vi "EOL Manual Controls.vi"(11 "main thread cluster":T1={"Application Status"="", "Switch Output Array"=[], "Switch Value Configuration"=[], "NVH Configuration"={"NVH Station?"=FALSE, "nvh app instance path"="", "NVH_ErrorMessages sv url"="", "NVH_Inputs sv url"="", "NVH_MotionNumber sv url"="", "NVH_Outputs sv url"="", "NVH_PartNumber sv url"="", "NVH_PartNumber_Echo sv url"="", "NVH_SerialNumber sv url"="", "NVH_AmbientTempF sv url"=""}, "rs232 port map"={"PMAC"="", "PS Port"="", "LVDT Unit"="", "RS232"=""}, "ethernet address map"={"LVDT 1 Unit"="172.17.53.143", "LVDT Unit 1 port"=0}, "paths"={"Base Path"=path "", "system error log path"=path "", "Error Table Path"=path "C/Labview Code/System/Error Table", "Store errors log path"=path "C/Labview Code/System/Error Table", "data bytes log path"=path "C/Labview Code/System/Error Table", "network path"=path "C/Labview Code/System/Error Table"}, "Station Index"=0, "Store Data"={"Motion Data Array"=[], "Error Table"=[], "Sun Shade Close Force Limits"={"Overall Min"=0.0, "Overall Max"=0.0, "Avg Min"=0.0, "Avg Max"=0.0, "Truncation Start"=0.0, "Truncation End"=0.0, "Variance"=0.0, "Check Noise"=FALSE}, "Sun Shade Open Force Limits"={"Overall Min"=0.0, "Overall Max"=0.0, "Avg Min"=0.0, "Avg Max"=0.0, "Truncation Start"=0.0, "Truncation End"=0.0, "Variance"=0.0, "Check Noise"=FALSE}, "Sunshade Open Data"=[], "Sunshade Close Data"=[], "Module Info"={"Serial Number"="", "Pallet Number"="", "Sunshade Color"="", "Inalfa Part Number"="", "Customer Number"=""}, "Sunsahde Close Raw Data"=[], "Sunshade Open Raw Data"=[], "Software Version"=[], "Constant Version"=[], "Hardware Version"=[], "Inalfa Part Number ECU"=[], "LVDT Data"=[], "Communication Line 1"=[], "Communication Line 2"=[], "Anti Pinch Force"=[], "Cycle Time"="", "Anti Pinch Vent Force"=[], "iGPS LVDT Data"=[], "data bytes log"=""}, "D in map"={"Abort Test"=enum."Dev2/port2/line6", "Start Test"=enum."Dev2/port2/line6"}, "DO Task"="station 1 dio", "ctl refs"={"Start Test"=refnum, "Abort Test"=refnum, "Manual Control"=refnum, "Route to Repair"=refnum, "Waveform Graph"=refnum, "Motion Data"=refnum, "all station status"=refnum, "Individual Station Status"=refnum, "exit program"=refnum, "Sunshade Servo Data Open"=refnum, "Sunshade Servo Data Close"=refnum, "Red-Rabbit Mode"=refnum, "Direct Manual Ctrl"=refnum}, "misc station config"={"Station Name"="", "is AT station?"=FALSE, "is audit station?"=FALSE, "power supply type"=enum."GENser", "use alt China TP2 LVDT Logic Seq"=FALSE, "hmi operator abort timeout"=0, "dump all analog values even if pass"=FALSE, "debug log pre-filter ap stream bytes"=FALSE, "use separate lvdt x and z extend tags"=FALSE, "is print"=FALSE}, "ethernet tcp refs"={"LVDT Unit"=refnum}, "Sunshade Barcode Scan"={"Sunshade Number 2"="", "Sunshade Number 1"="", "Keyence tuning bank idx"=0}, "AP Test Data"={"Raw Sunshade AP Data"="", "Raw Glass AP Data"="", "PMAC Read Counter"=0.0, "Database AP Data"=[]}, "Motion Status"={"hmi operator abort start time"=0, "Current Data Index"=0, "Analog Data"=[], "Motor Position Hex"=0, "Messages Index"=0, "Last Bytes"=[], "Current Hall Position"=0, "Motion Stop Timer"=0, "Position Test"=enum."Not Tested", "Noise Test"=enum."Not Tested", "motion stop check initialized"=FALSE, "remote sense enabled"=FALSE, "Motion"=enum."Glass Teach"}, "LVDT Status"={"LVDT's stored config"=[], "lvdt precision"={"truncate instead of rounding"=FALSE, "decimal places"=0}}, "Sequence State"={"Step Description"="", "Cycle Start Time"=0, "Step Data String"="", "Pass?"=FALSE, "Seqence"=[], "Active Step"=0, "Testing?"=FALSE, "Red-Rabbit Mode"=FALSE, "route-to-repair mode"=FALSE, "NVH Status"={"Restart IRQ Counter"=0, "NVH Test Needed?"=FALSE, "NVH Test Running?"=FALSE}, "Present (s)"=0.0, "Hold Mode?"=FALSE, "Hold?"=FALSE, "Rx Invalid?"=FALSE}, "misc status"={"delay start time (ticks)"=0, "In Vehicle Mode?"=FALSE, "Diag Mode?"=FALSE, "Serial Port Configured?"=FALSE, "PS Voltage"=0.0, "Diag Serial Port"="", "Part Setup"={"Communication Type"=enum."None", "Send Messages to"=enum."Glass", "RAP Signal"=enum."High", "Motor Type"=enum."Smart Motor", "NVH Part Number"=0, "Turn Off Timer"=0, "Part Type"=""}, "Part History Number"="", "Plant Number"=0, "AP Data Type"=enum."91/61", "Real Rollo?"=FALSE}, "NVH Operator?"=FALSE, "NVH Pass?"=FALSE, "Operator Pass?"=FALSE, "Operator Action?"=FALSE, "Noise Source"=0, "USBHandle"=0, "PeakInfo"="", "PeakNumber"=0, "NVH Motion Steps"=[], "Second Check?"=FALSE, "Decibel data"=[], "Direct Control Info"={"EnableStopOnHome"=FALSE, "EnableStopOnPos"=FALSE, "TeachEvent"=FALSE, "open offset"=0, "close offset"=0, "Derect control"=FALSE, "set position"=[], "teach pass "=FALSE, "Drift offsets"=[], "Hall Positions"=[]}, "manual control(direct)"=FALSE, "LIN INFO"={"Toolkit Type"=enum."Inalfa LIN", "NAD"=36, "Inalfa LIN"={"Master Frame(3C)"="", "Slave Frame(3D)"="NIXNET_exampleLDF", "Request Schedule"="NIXNET_exampleLDF", "Response Schedule"="CEMLIN3DiagResponseSchedule\nSPA3414_ConfigurationsCMAGeely_CEMCALYPSOSDB34XX0Cfg_LIN3_190709_", "Frame Write SCU"="", "Frame Read SCU"="", "LIN Name"=""}, "ADCS LIN"={"Port"="MasterReq\nSPA3414_ConfigurationsCMAGeely_CEMCALYPSOSDB34XX0Cfg_LIN3_190709_", "HW select"=0, "XNET Cluster"="SlaveResp\nSPA3414_ConfigurationsCMAGeely_CEMCALYPSOSDB34XX0Cfg_LIN3_190709_", "ByteCmd Path"=path "C/Labview Code/System/ByteCmdConfig.txt"}, "TS LIN"={"ref info"=refnum, "LIN Channel"=0, "ByteCmd Path"=path "C/Labview Code/System/ByteCmdConfig.txt"}}, "Config Info"=variant} {"LIN INFO"."NAD" format="%.0x"; "LIN INFO"."ADCS LIN"."HW select" items=["NI-XNET", "NI-CAN"]; "LVDT Status"."LVDT's stored config"."Lower Limit" format="%.2f"; "LVDT Status"."LVDT's stored config"."Upper Limit" format="%.2f"; "Store Data"."Sun Shade Open Force Limits"."Variance" format="%.2g"; "Store Data"."Sun Shade Open Force Limits"."Truncation End" format="%.2g"; "Store Data"."Sun Shade Open Force Limits"."Truncation Start" format="%.2g"; "Store Data"."Sun Shade Open Force Limits"."Avg Max" format="%.2g"; "Store Data"."Sun Shade Open Force Limits"."Avg Min" format="%.2g"; "Store Data"."Sun Shade Open Force Limits"."Overall Max" format="%.2g"; "Store Data"."Sun Shade Open Force Limits"."Overall Min" format="%.2g"; "Store Data"."Sun Shade Close Force Limits"."Variance" format="%.2g"; "Store Data"."Sun Shade Close Force Limits"."Truncation End" format="%.2g"; "Store Data"."Sun Shade Close Force Limits"."Truncation Start" format="%.2g"; "Store Data"."Sun Shade Close Force Limits"."Avg Max" format="%.2g"; "Store Data"."Sun Shade Close Force Limits"."Avg Min" format="%.2g"; "Store Data"."Sun Shade Close Force Limits"."Overall Max" format="%.2g"; "Store Data"."Sun Shade Close Force Limits"."Overall Min" format="%.2g"; "Store Data"."Motion Data Array"."Motion Data Limits"."LIN Msg"."Msg" format="%02x"; "Store Data"."Motion Data Array"."Motion Data Limits"."LIN Msg"."ID" format="%02x"}) -> (3 "main thread cluster out":T1={"Application Status"="", "Switch Output Array"=[], "Switch Value Configuration"=[], "NVH Configuration"={"NVH Station?"=FALSE, "nvh app instance path"="", "NVH_ErrorMessages sv url"="", "NVH_Inputs sv url"="", "NVH_MotionNumber sv url"="", "NVH_Outputs sv url"="", "NVH_PartNumber sv url"="", "NVH_PartNumber_Echo sv url"="", "NVH_SerialNumber sv url"="", "NVH_AmbientTempF sv url"=""}, "rs232 port map"={"PMAC"="", "PS Port"="", "LVDT Unit"="", "RS232"=""}, "ethernet address map"={"LVDT 1 Unit"="172.17.53.143", "LVDT Unit 1 port"=0}, "paths"={"Base Path"=path "", "system error log path"=path "", "Error Table Path"=path "C/Labview Code/System/Error Table", "Store errors log path"=path "C/Labview Code/System/Error Table", "data bytes log path"=path "C/Labview Code/System/Error Table", "network path"=path "C/Labview Code/System/Error Table"}, "Station Index"=0, "Store Data"={"Motion Data Array"=[], "Error Table"=[], "Sun Shade Close Force Limits"={"Overall Min"=0.0, "Overall Max"=0.0, "Avg Min"=0.0, "Avg Max"=0.0, "Truncation Start"=0.0, "Truncation End"=0.0, "Variance"=0.0, "Check Noise"=FALSE}, "Sun Shade Open Force Limits"={"Overall Min"=0.0, "Overall Max"=0.0, "Avg Min"=0.0, "Avg Max"=0.0, "Truncation Start"=0.0, "Truncation End"=0.0, "Variance"=0.0, "Check Noise"=FALSE}, "Sunshade Open Data"=[], "Sunshade Close Data"=[], "Module Info"={"Serial Number"="", "Pallet Number"="", "Sunshade Color"="", "Inalfa Part Number"="", "Customer Number"=""}, "Sunsahde Close Raw Data"=[], "Sunshade Open Raw Data"=[], "Software Version"=[], "Constant Version"=[], "Hardware Version"=[], "Inalfa Part Number ECU"=[], "LVDT Data"=[], "Communication Line 1"=[], "Communication Line 2"=[], "Anti Pinch Force"=[], "Cycle Time"="", "Anti Pinch Vent Force"=[], "iGPS LVDT Data"=[], "data bytes log"=""}, "D in map"={"Abort Test"=enum."Dev2/port2/line6", "Start Test"=enum."Dev2/port2/line6"}, "DO Task"="station 1 dio", "ctl refs"={"Start Test"=refnum, "Abort Test"=refnum, "Manual Control"=refnum, "Route to Repair"=refnum, "Waveform Graph"=refnum, "Motion Data"=refnum, "all station status"=refnum, "Individual Station Status"=refnum, "exit program"=refnum, "Sunshade Servo Data Open"=refnum, "Sunshade Servo Data Close"=refnum, "Red-Rabbit Mode"=refnum, "Direct Manual Ctrl"=refnum}, "misc station config"={"Station Name"="", "is AT station?"=FALSE, "is audit station?"=FALSE, "power supply type"=enum."GENser", "use alt China TP2 LVDT Logic Seq"=FALSE, "hmi operator abort timeout"=0, "dump all analog values even if pass"=FALSE, "debug log pre-filter ap stream bytes"=FALSE, "use separate lvdt x and z extend tags"=FALSE, "is print"=FALSE}, "ethernet tcp refs"={"LVDT Unit"=refnum}, "Sunshade Barcode Scan"={"Sunshade Number 2"="", "Sunshade Number 1"="", "Keyence tuning bank idx"=0}, "AP Test Data"={"Raw Sunshade AP Data"="", "Raw Glass AP Data"="", "PMAC Read Counter"=0.0, "Database AP Data"=[]}, "Motion Status"={"hmi operator abort start time"=0, "Current Data Index"=0, "Analog Data"=[], "Motor Position Hex"=0, "Messages Index"=0, "Last Bytes"=[], "Current Hall Position"=0, "Motion Stop Timer"=0, "Position Test"=enum."Not Tested", "Noise Test"=enum."Not Tested", "motion stop check initialized"=FALSE, "remote sense enabled"=FALSE, "Motion"=enum."Glass Teach"}, "LVDT Status"={"LVDT's stored config"=[], "lvdt precision"={"truncate instead of rounding"=FALSE, "decimal places"=0}}, "Sequence State"={"Step Description"="", "Cycle Start Time"=0, "Step Data String"="", "Pass?"=FALSE, "Seqence"=[], "Active Step"=0, "Testing?"=FALSE, "Red-Rabbit Mode"=FALSE, "route-to-repair mode"=FALSE, "NVH Status"={"Restart IRQ Counter"=0, "NVH Test Needed?"=FALSE, "NVH Test Running?"=FALSE}, "Present (s)"=0.0, "Hold Mode?"=FALSE, "Hold?"=FALSE, "Rx Invalid?"=FALSE}, "misc status"={"delay start time (ticks)"=0, "In Vehicle Mode?"=FALSE, "Diag Mode?"=FALSE, "Serial Port Configured?"=FALSE, "PS Voltage"=0.0, "Diag Serial Port"="", "Part Setup"={"Communication Type"=enum."None", "Send Messages to"=enum."Glass", "RAP Signal"=enum."High", "Motor Type"=enum."Smart Motor", "NVH Part Number"=0, "Turn Off Timer"=0, "Part Type"=""}, "Part History Number"="", "Plant Number"=0, "AP Data Type"=enum."91/61", "Real Rollo?"=FALSE}, "NVH Operator?"=FALSE, "NVH Pass?"=FALSE, "Operator Pass?"=FALSE, "Operator Action?"=FALSE, "Noise Source"=0, "USBHandle"=0, "PeakInfo"="", "PeakNumber"=0, "NVH Motion Steps"=[], "Second Check?"=FALSE, "Decibel data"=[], "Direct Control Info"={"EnableStopOnHome"=FALSE, "EnableStopOnPos"=FALSE, "TeachEvent"=FALSE, "open offset"=0, "close offset"=0, "Derect control"=FALSE, "set position"=[], "teach pass "=FALSE, "Drift offsets"=[], "Hall Positions"=[]}, "manual control(direct)"=FALSE, "LIN INFO"={"Toolkit Type"=enum."Inalfa LIN", "NAD"=36, "Inalfa LIN"={"Master Frame(3C)"="", "Slave Frame(3D)"="NIXNET_exampleLDF", "Request Schedule"="NIXNET_exampleLDF", "Response Schedule"="CEMLIN3DiagResponseSchedule\nSPA3414_ConfigurationsCMAGeely_CEMCALYPSOSDB34XX0Cfg_LIN3_190709_", "Frame Write SCU"="", "Frame Read SCU"="", "LIN Name"=""}, "ADCS LIN"={"Port"="MasterReq\nSPA3414_ConfigurationsCMAGeely_CEMCALYPSOSDB34XX0Cfg_LIN3_190709_", "HW select"=0, "XNET Cluster"="SlaveResp\nSPA3414_ConfigurationsCMAGeely_CEMCALYPSOSDB34XX0Cfg_LIN3_190709_", "ByteCmd Path"=path "C/Labview Code/System/ByteCmdConfig.txt"}, "TS LIN"={"ref info"=refnum, "LIN Channel"=0, "ByteCmd Path"=path "C/Labview Code/System/ByteCmdConfig.txt"}}, "Config Info"=variant} {"LIN INFO"."NAD" format="%.0x"; "LIN INFO"."ADCS LIN"."HW select" items=["NI-XNET", "NI-CAN"]; "LVDT Status"."LVDT's stored config"."Lower Limit" format="%.2f"; "LVDT Status"."LVDT's stored config"."Upper Limit" format="%.2f"; "Store Data"."Sun Shade Open Force Limits"."Variance" format="%.2g"; "Store Data"."Sun Shade Open Force Limits"."Truncation End" format="%.2g"; "Store Data"."Sun Shade Open Force Limits"."Truncation Start" format="%.2g"; "Store Data"."Sun Shade Open Force Limits"."Avg Max" format="%.2g"; "Store Data"."Sun Shade Open Force Limits"."Avg Min" format="%.2g"; "Store Data"."Sun Shade Open Force Limits"."Overall Max" format="%.2g"; "Store Data"."Sun Shade Open Force Limits"."Overall Min" format="%.2g"; "Store Data"."Sun Shade Close Force Limits"."Variance" format="%.2g"; "Store Data"."Sun Shade Close Force Limits"."Truncation End" format="%.2g"; "Store Data"."Sun Shade Close Force Limits"."Truncation Start" format="%.2g"; "Store Data"."Sun Shade Close Force Limits"."Avg Max" format="%.2g"; "Store Data"."Sun Shade Close Force Limits"."Avg Min" format="%.2g"; "Store Data"."Sun Shade Close Force Limits"."Overall Max" format="%.2g"; "Store Data"."Sun Shade Close Force Limits"."Overall Min" format="%.2g"; "Store Data"."Motion Data Array"."Motion Data Limits"."LIN Msg"."Msg" format="%02x"; "Store Data"."Motion Data Array"."Motion Data Limits"."LIN Msg"."ID" format="%02x"})   [LabVIEW 2018]
uses:
  02.Type Def's/debug io digital io.ctl
  02.Type Def's/EOL Analog Input Control.ctl
  05.UserVI's/type defs/EOL LVDT's Check Controller.ctl
  02.Type Def's/main state cluster.ctl
  02.Type Def's/All Switch Configuration Cluster.ctl
  02.Type Def's/All Motions.ctl
  02.Type Def's/EOL Switch Value Configuration Cluster.ctl
  02.Type Def's/EOL Switch Max Min Check Cluster.ctl
  02.Type Def's/station nvh config.ctl
  02.Type Def's/station rs232 port map.ctl
  02.Type Def's/station ethernet address map.ctl
  02.Type Def's/station paths.ctl
  02.Type Def's/EOL Save Module Test Data Control.ctl
  02.Type Def's/EOL Motion Database Table.ctl
  05.UserVI's/type defs/17x Audit Motion Data Seq Control.ctl
  05.UserVI's/type defs/17x AP Data Type.ctl
  05.UserVI's/type defs/17x Sunshade Limts Seq.ctl
  02.Type Def's/EOL Module Info Control.ctl
  02.Type Def's/station DI map.ctl
  05.UserVI's/type defs/EOL Global Digital Input Control.ctl
  02.Type Def's/control refs.ctl
  02.Type Def's/station motion data indicator.ctl
  02.Type Def's/Screen Motion Data.ctl
  02.Type Def's/Pass Fail Control.ctl
  02.Type Def's/station hmi.ctl
  02.Type Def's/lvdt name val pair.ctl
  02.Type Def's/individual station status.ctl
  02.Type Def's/misc station config.ctl
  05.UserVI's/Lambda Power/power supply types.ctl
  05.UserVI's/LVDT's/lvdt precision.ctl
  02.Type Def's/sequence state.ctl
  05.UserVI's/sequence/type defs/Sequence Info.ctl
  05.UserVI's/type defs/EOL Part Setup.ctl
  02.Type Def's/All Communication Types.ctl
  05.UserVI's/type defs/Communication with Motors.ctl
  05.UserVI's/type defs/RAP Signal Control.ctl
  05.UserVI's/type defs/EOL Motor Type.ctl
  02.Type Def's/station LIN config.ctl
  03.Inalfa LIN/LIN Device.ctl
  <vilib>/CMC.AME/Inalfa ADCS/Ctl'Def/ADCS_LIN info.ctl
  C:/Program Files (x86)/National Instruments/LabVIEW 2018/vi.lib/CMC.AME/Inalfa TS LIN/TOSUN/TSMaster/bin/Interop.TSMasterAPI.dll
  Program Files (x86)/National Instruments/LabVIEW 2018/vi.lib/CMC.AME/Inalfa TS LIN/TOSUN/TSMaster/bin/Interop.TSMasterAPI.dll
  06.Test Loop/Sub'VIs/Type Def's/Config Info.ctl
  03.Inalfa LIN/LIN sequence for self SCU.ctl
  05.UserVI's/type defs/EOL Global Digital Output Cluster Control.ctl
  05.UserVI's/type defs/EOL Global Digital Output Control.ctl
  05.UserVI's/BarCode/typedefs/barcode format params.ctl
  05.UserVI's/BarCode/typedefs/barcode printer types.ctl
  03.Inalfa LIN/LIN show messages.ctl
  <vilib>/Utility/config.llb/Read Key (String).vi
  <vilib>/Utility/config.llb/Write Key (String).vi
  <vilib>/Instr/_visa.llb/VISA Configure Serial Port (Instr).vi
  <vilib>/Utility/file.llb/Write To Spreadsheet File (string).vi
  <vilib>/Utility/file.llb/Read From Spreadsheet File (string).vi
  <vilib>/Utility/config.llb/NI_LVConfig.lvlib
  <resource>/objmgr/daqmx.rc
panel:
  out "错误输出":errorcluster
  in  "Exit":bool
  out "Title":string="Manual Control"
  in  "Tab Control 3":T35(tab)=enum."Barcode Read and Print"
  in  "Sunroof Operation":bool
  in  "Re-Init PS":bool
  out "All Inputs":T36[](array[typedef])=[{"channel name"="Abort Test", "state"=FALSE}, {"channel name"="Start Test", "state"=FALSE}]
  in  "Set Voltage":bool
  in  "Output Voltage":dbl=13.5
  out "Audit Graph":sgl[][](graph)
  in  "Analog Control":T37
  in  "Analog Control 2":T37=enum."Motor Current"
  in  "Analog Control 3":T37=enum."Switch A"
  in  "Color Box 10":u32(colorbox)=16860
  in  "Color Box 11":u32(colorbox)=16711680
  in  "Color Box 12":u32(colorbox)
  in  "Digital Output Array":T36[](array[typedef])=[{"channel name"="Comm Power", "state"=FALSE}, {"channel name"="Switch 1", "state"=FALSE}, {"channel name"="Switch 2", "state"=FALSE}, {"channel name"="Switch 3", "state"=FALSE}, {"channel name"="Switch 4", "state"=FALSE}, {"channel name"="Switch 5", "state"=FALSE}, {"channel name"="Switch 6", "state"=FALSE}, {"channel name"="Glass Analog Switch 1", "state"=FALSE}, {"channel name"="Glass Analog Switch 2", "state"=FALSE}, {"channel name"="Glass Analog Switch 3", "state"=FALSE}, {"channel name"="Glass Analog Switch 4", "state"=FALSE}, {"channel name"="Glass Motor Relay 1", "state"=FALSE}, {"channel name"="Glass Motor Relay 2", "state"=FALSE}, {"channel name"="Sunshade Motor Relay 1", "state"=FALSE}, {"channel name"="Sunshade Motor Relay 2", "state"=FALSE}, {"channel name"="Ignition High", "state"=FALSE}, {"channel name"="Ignition Low", "state"=FALSE}, {"channel name"="Battery", "state"=FALSE}, {"channel name"="Sunshade Analog Switch 1", "state"=FALSE}, {"channel name"="Sunshade Analog Switch 2", "state"=FALSE}, {"channel name"="Sunshade Analog Switch 3", "state"=FALSE}, {"channel name"="Sunshade Analog Switch 4", "state"=FALSE}, {"channel name"="NI LIN", "state"=FALSE}, {"channel name"="RS232 LIN", "state"=FALSE}, {"channel name"="RS232", "state"=FALSE}, {"channel name"="CAN", "state"=FALSE}, {"channel name"="Park/Enable", "state"=FALSE}]
  out "Communications Tab":enum32{"Send Message"}(tab)
  out "Hold？":bool
  in  "Multicolumn Listbox":i32(listbox)
  in  "Part Type":u16(ring) items=["OE", "EX1H", "EX1E"]
  in  "Send Inalfa SCU Message":bool
  in  "Choose Sequence":T38
  out "LIN show Tags":T39(tab)
  in  "Vent Cycles":u16
  in  "Slide Cycles":u16
  out "slide cycle":u16
  out "Software Level":string
  out "Hardware Level":string
  out "Calfile Level":string
  in  "Tx3":u8[][](array[numeric]) format="%02x"
  in  "Tx2":u8[][](array[numeric]) format="%02x"
  in  "Rx2":u8[](array[numeric]) format="%02x"
  in  "Position":u16
  out "glass position":u16
  out "sunshade position":u16
  in  "BYD Teach":string
  out "Recive？":bool
  in  "Send Message":bool
  in  "Message List":i32(listbox)
  out "Toolkit Type":enum16{"Inalfa LIN", "ADCS LIN", "TS LIN"}(ring)=enum."ADCS LIN"
  out "String":string
  out "RSLinx Read Boolean":cluster{"Tag String":string, "Boolean":bool}[](array[cluster])=[{"Tag String"="", "Boolean"=FALSE}, {"Tag String"="", "Boolean"=FALSE}, {"Tag String"="", "Boolean"=FALSE}, {"Tag String"="", "Boolean"=FALSE}, {"Tag String"="", "Boolean"=FALSE}, {"Tag String"="", "Boolean"=FALSE}, {"Tag String"="", "Boolean"=FALSE}, {"Tag String"="", "Boolean"=FALSE}, {"Tag String"="", "Boolean"=FALSE}, {"Tag String"="", "Boolean"=FALSE}, {"Tag String"="", "Boolean"=FALSE}, {"Tag String"="S101.PXI.Signals.Mounting_Bolts.MountBoltSnsr01", "Boolean"=FALSE}, {"Tag String"="S101.PXI.Signals.Mounting_Bolts.MountBoltSnsr02", "Boolean"=FALSE}, {"Tag String"="S101.PXI.Signals.Mounting_Bolts.MountBoltSnsr03", "Boolean"=FALSE}, {"Tag String"="S101.PXI.Signals.Mounting_Bolts.MountBoltSnsr04", "Boolean"=FALSE}, {"Tag String"="S101.PXI.Signals.Mounting_Bolts.MountBoltSnsr05", "Boolean"=FALSE}, {"Tag String"="S101.PXI.Signals.Mounting_Bolts.MountBoltSnsr06", "Boolean"=FALSE}, {"Tag String"="S101.PXI.Signals.Mounting_Bolts.MountBoltSnsr07", "Boolean"=FALSE}, {"Tag String"="S101.PXI.Signals.Mounting_Bolts.MountBoltSnsr08", "Boolean"=FALSE}, {"Tag String"="S101.PXI.Signals.Mounting_Bolts.MountBoltSnsr09", "Boolean"=FALSE}, {"Tag String"="S101.PXI.Signals.Mounting_Bolts.MountBoltSnsr10", "Boolean"=FALSE}, {"Tag String"="S101.PXI.Signals.Mounting_Bolts.MountBoltSnsr11", "Boolean"=FALSE}, {"Tag String"="S101.PXI.Signals.Mounting_Bolts.MountBoltSnsr12", "Boolean"=FALSE}, {"Tag String"="S101.PXI.Signals.Mounting_Bolts.MountBoltSnsr13", "Boolean"=FALSE}, {"Tag String"="S101.PXI.Signals.Mounting_Bolts.MountBoltSnsr14", "Boolean"=FALSE}, {"Tag String"="S101.PXI.Signals.Mounting_Bolts.MountBoltSnsr15", "Boolean"=FALSE}, {"Tag String"="S101.PXI.Signals.Mounting_Bolts.MountBoltSnsr16", "Boolean"=FALSE}, {"Tag String"="S101.PXI.Signals.Mounting_Bolts.MountBoltSnsr17", "Boolean"=FALSE}, {"Tag String"="S101.PXI.Signals.Mounting_Bolts.MountBoltSnsr18", "Boolean"=FALSE}, {"Tag String"="S101.PXI.Signals.Mounting_Bolts.MountBoltSnsr19", "Boolean"=FALSE}, {"Tag String"="S101.PXI.Signals.Mounting_Bolts.MountBoltSnsr20", "Boolean"=FALSE}, {"Tag String"="S101.PXI.Signals.Mounting_Bolts.MountBoltSnsr21", "Boolean"=FALSE}, {"Tag String"="S101.PXI.Signals.StartTest", "Boolean"=FALSE}, {"Tag String"="S101.PXI.Signals.AbortTest", "Boolean"=FALSE}, {"Tag String"="", "Boolean"=FALSE}, {"Tag String"="", "Boolean"=FALSE}, {"Tag String"="S101.PXI.Signals.SoundTestAbort", "Boolean"=FALSE}, {"Tag String"="S101.PXI.Signals.BCData.Print", "Boolean"=FALSE}, {"Tag String"="", "Boolean"=FALSE}, {"Tag String"="", "Boolean"=FALSE}, {"Tag String"="", "Boolean"=FALSE}, {"Tag String"="", "Boolean"=FALSE}]
  out "RSLinx Read String":cluster{"Tag String":string, "String":string}[](array[cluster])=[{"Tag String"="", "String"=""}, {"Tag String"="", "String"="0"}, {"Tag String"="", "String"=""}, {"Tag String"="", "String"=""}, {"Tag String"="", "String"=""}, {"Tag String"="", "String"=""}, {"Tag String"="", "String"=""}, {"Tag String"="", "String"=""}, {"Tag String"="S101.PXI.Signals.PlltData.Sunshade2", "String"=""}, {"Tag String"="S101.PXI.Signals.BCData.SN", "String"="1234"}, {"Tag String"="S101.PXI.Signals.BCData.PN", "String"="1234"}, {"Tag String"="S101.PXI.Signals.BCData.Color", "String"="red"}, {"Tag String"="S101.PXI.Signals.BCData.Model", "String"="1234"}, {"Tag String"="S101.PXI.Signals.BCData.CN", "String"="5678"}, {"Tag String"="S101.PXI.Signals.BCData.PHN", "String"="5678"}]
  in  "RSLinx Write Tag String Array Data":string[](array[string])=["", "", "", "", "", "", "", "", "", "", ""]
  out "RSLinx Write Tag String Array Names":string[](array[string])
  out "RSLinx Write Tag Boolean Array Names":string[](array[string])
  in  "RSLinx Write Tag Boolean Array Data":bool[](array[boolean])=[FALSE, FALSE, FALSE, FALSE, FALSE, FALSE, FALSE, FALSE, FALSE, FALSE]
  in  "Barcode Print Part Type":u16(ring) items=["OE", "EX1H", "EX1E"]
  in  "Barcode Print Part Type":u16(ring) items=["OE", "EX1H", "EX1E"]
  in  "Scan Audit Station Barcode 2 (ss)":bool
  in  "Line Number":u8 max=9
  in  "Customer Name:":string="BMW"
  in  "PHN:":string
  in  "Customer Number:":string="805902507"
  in  "Part Type:":string
  in  "Print Audit St 2D Barcode":bool
  in  "Sunshade Color":string="Reptile Anthraite Black"
  in  "IRS Number:":string="30022369F"
  in  "Serial Number:":string="00103142014"
  in  "Scan Audit Station Barcode":bool
  in  "Scan Station 50 Sunshade Barcode":bool
  in  "TLL/PHN":string="70"
  in  "Color Name":string="REPTILE ANTHRACITE"
  in  "Inalfa Part Number":string="30022369F"
  in  "Module Serial Number":string="00103142014"
  in  "Customer Number":string="805902507"
  in  "Print Station 60 Barcode":bool
  in  "LVDT Part Type":u16(ring) items=["OE", "EX1H", "EX1E"]
  in  "LVDT's Write Preset Data":bool
  in  "LVDT's Read Preset Data":bool
  in  "LVDT's Read Data":bool
  in  "LVDT's Write Data":bool
  in  "LVDT's Limit Array":T22[](array[typedef])=[{"Upper Limit"=1.0, "Lower Limit"=-1.0, "LVDT Name"="LVDT 1", "Check"=FALSE}, {"Upper Limit"=1.0, "Lower Limit"=-1.0, "LVDT Name"="LVDT 2", "Check"=FALSE}, {"Upper Limit"=1.0, "Lower Limit"=-1.0, "LVDT Name"="LVDT 3", "Check"=FALSE}, {"Upper Limit"=1.0, "Lower Limit"=-1.0, "LVDT Name"="LVDT 4", "Check"=FALSE}, {"Upper Limit"=1.0, "Lower Limit"=-1.0, "LVDT Name"="LVDT 5", "Check"=FALSE}, {"Upper Limit"=1.0, "Lower Limit"=-1.0, "LVDT Name"="LVDT 6", "Check"=FALSE}, {"Upper Limit"=1.0, "Lower Limit"=-1.0, "LVDT Name"="LVDT 7", "Check"=FALSE}, {"Upper Limit"=1.0, "Lower Limit"=-1.0, "LVDT Name"="LVDT 8", "Check"=FALSE}, {"Upper Limit"=1.0, "Lower Limit"=-1.0, "LVDT Name"="LVDT 9", "Check"=FALSE}, {"Upper Limit"=1.0, "Lower Limit"=-1.0, "LVDT Name"="LVDT 10", "Check"=FALSE}, {"Upper Limit"=1.0, "Lower Limit"=-1.0, "LVDT Name"="LVDT 11", "Check"=FALSE}, {"Upper Limit"=1.0, "Lower Limit"=-1.0, "LVDT Name"="LVDT 12", "Check"=FALSE}, {"Upper Limit"=1.0, "Lower Limit"=-1.0, "LVDT Name"="LVDT 13", "Check"=FALSE}, {"Upper Limit"=1.0, "Lower Limit"=-1.0, "LVDT Name"="LVDT 14", "Check"=FALSE}, {"Upper Limit"=1.0, "Lower Limit"=-1.0, "LVDT Name"="LVDT 15", "Check"=FALSE}] {"Lower Limit" format="%.2f"; "Upper Limit" format="%.2f"}
  in  "truncate instead of round":bool
  in  "Desired Decimal Points":u8=2
  out "rs232 port map":T7
  out "Reading Count":dbl
  in  "Clear PMAC Buffer":bool
  out "PMAC Reading":string
  in  "Read PMAC":bool
  out "PMAC Reading 2":string
  # "Sunroof Barcode"
  # "Pallet Number"
  # "Part Type"
  # "Application Status"
  # "Current Step"
  # "Cycle Time"
  # "Pass / Fail"
  # "Shade Close"
  # "Actual Data"
  # "Limits"
  # "Avg Current"
  # "Run Time"
  # "Speed"
  # "Noise Test"
  # "Position"
  # "Shade Open"
  # "Actual Data"
  # "Limits"
  # "Avg Current"
  # "Run Time"
  # "Speed"
  # "Noise Test"
  # "Position"
  # "Vent Close"
  # "Actual Data"
  # "Limits"
  # "Avg Current"
  # "Run Time"
  # "Speed"
  # "Noise Test"
  # "Position"
  # "Vent Open"
  # "Actual Data"
  # "Limits"
  # "Avg Current"
  # "Run Time"
  # "Speed"
  # "Noise Test"
  # "Position"
  # "Slide Close"
  # "Actual Data"
  # "Limits"
  # "Avg Current"
  # "Run Time"
  # "Speed"
  # "Noise Test"
  # "Position"
  # "Slide Open"
  # "Actual Data"
  # "Limits"
  # "Avg Current"
  # "Run Time"
  # "Speed"
  # "Noise Test"
  # "Position"
  # "Min"
  # "N"
  # "Min"
  # "Start"
  # "N"
  # "Max"
  # "N"
  # "Max"
  # "N"
  # "End"
  # "Min"
  # "N"
  # "Min"
  # "Start"
  # "N"
  # "Max"
  # "N"
  # "Max"
  # "N"
  # "End"
  # "Min"
  # "Max"
  # "Sunroof Barcode"
  # "Pallet Number"
  # "Part Type"
  # "Application Status"
  # "Current Step"
  # "Cycle Time"
  # "Pass / Fail"
  # "Shade Close"
  # "Actual Data"
  # "Limits"
  # "Avg Current"
  # "Run Time"
  # "Speed"
  # "Noise Test"
  # "Position"
  # "Shade Open"
  # "Actual Data"
  # "Limits"
  # "Avg Current"
  # "Run Time"
  # "Speed"
  # "Noise Test"
  # "Position"
  # "Vent Close"
  # "Actual Data"
  # "Limits"
  # "Avg Current"
  # "Run Time"
  # "Speed"
  # "Noise Test"
  # "Position"
  # "Vent Open"
  # "Actual Data"
  # "Limits"
  # "Avg Current"
  # "Run Time"
  # "Speed"
  # "Noise Test"
  # "Position"
  # "Slide Close"
  # "Actual Data"
  # "Limits"
  # "Avg Current"
  # "Run Time"
  # "Speed"
  # "Noise Test"
  # "Position"
  # "Slide Open"
  # "Actual Data"
  # "Limits"
  # "Avg Current"
  # "Run Time"
  # "Speed"
  # "Noise Test"
  # "Position"
  # "Min"
  # "N"
  # "Min"
  # "Start"
  # "N"
  # "Max"
  # "N"
  # "Max"
  # "N"
  # "End"
  # "Min"
  # "N"
  # "Min"
  # "Start"
  # "N"
  # "Max"
  # "N"
  # "Max"
  # "N"
  # "End"
  # "Min"
  # "Max"
  # "DO"
  # "DI"
  # "Barcode Printing Station"
  # "Audit Station"
  # "LVDT Name"
  # "Current Value"
  # "Preset"
  # "Preset?"
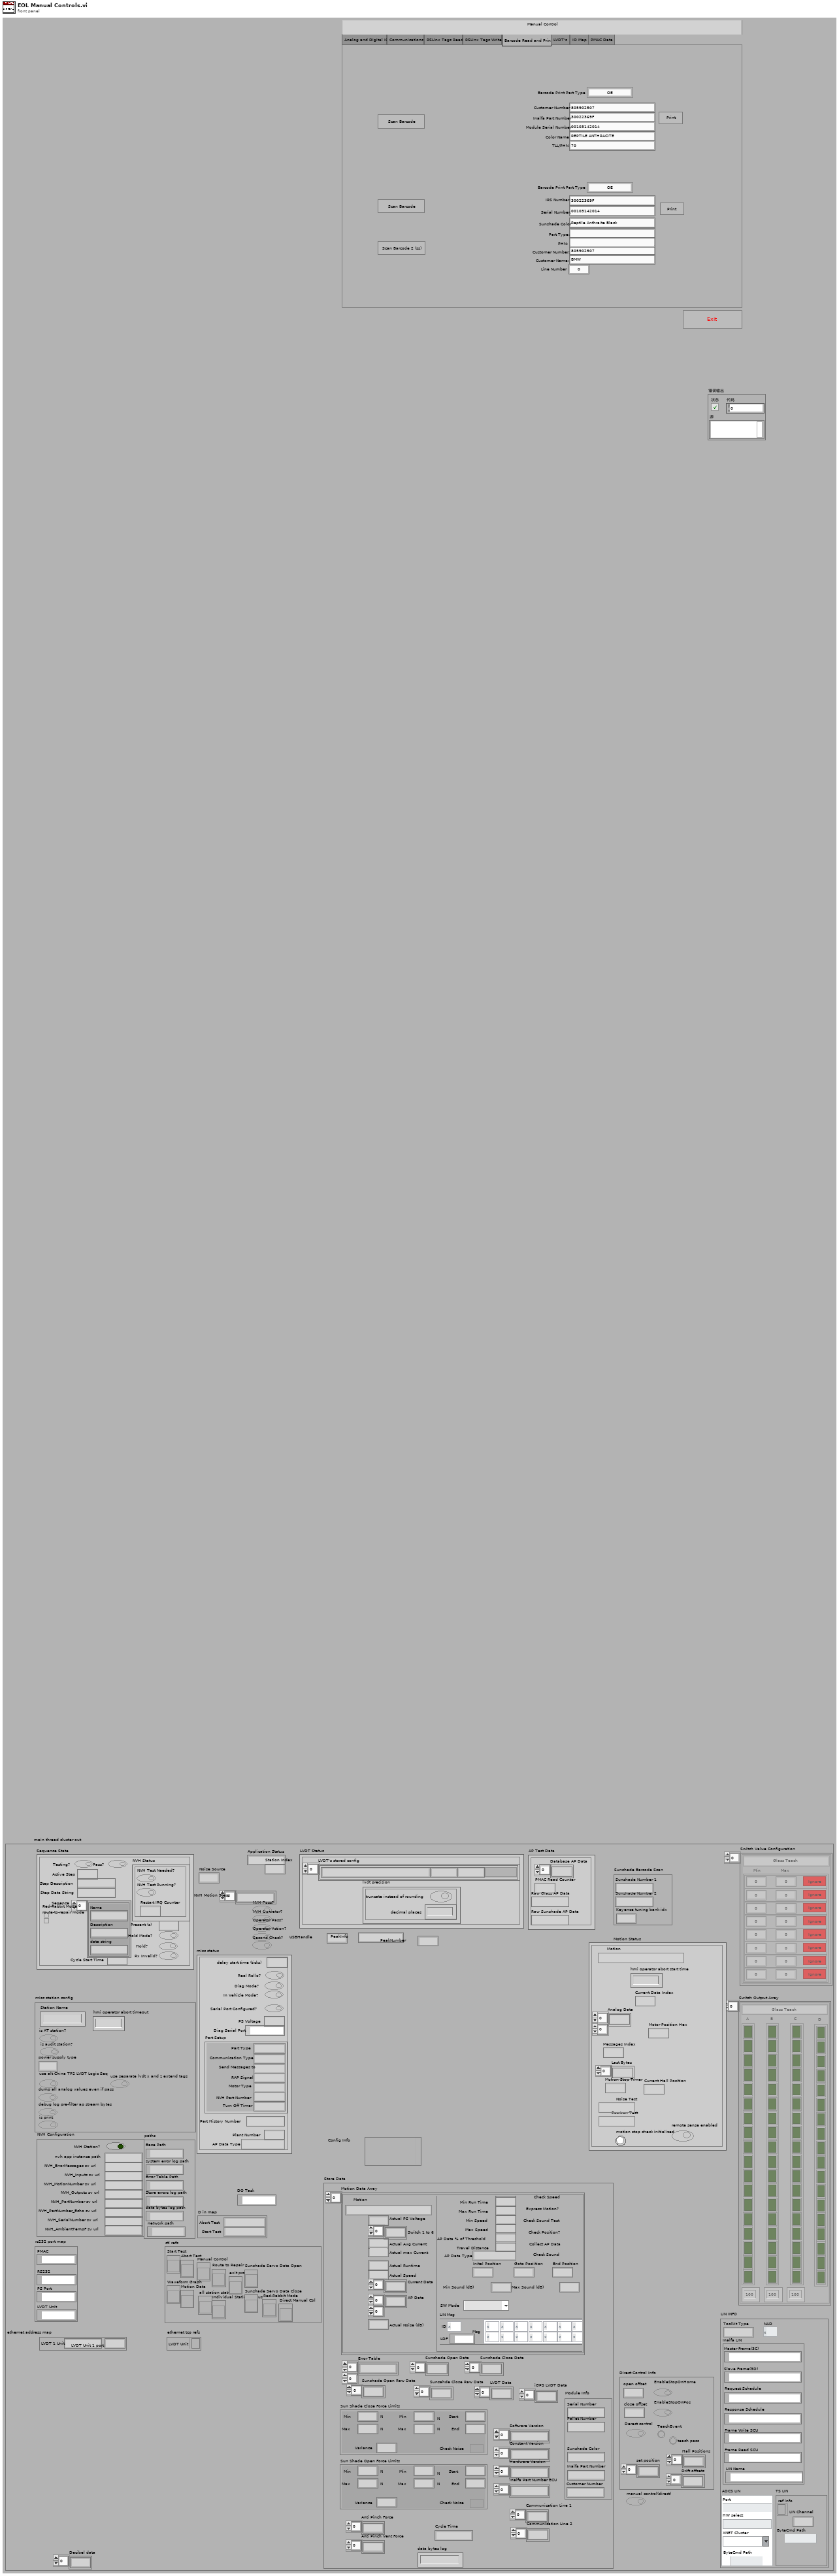
[diagram p1: front panel]
types:
  T1 = typedef "main state cluster.ctl" = cluster{"Application Status":string, "Switch Output Array":T2[], "Switch Value Configuration":T4[], "NVH Configuration":T6, "rs232 port map":T7, "ethernet address map":T8, "paths":T9, "Station Index":i32, "Store Data":T10, "D in map":T16, "DO Task":refnum<k21>, "ctl refs":T18, "misc station config":T19, "ethernet tcp refs":cluster{"LVDT Unit":refnum<k5>}, "Sunshade Barcode Scan":cluster{"Sunshade Number 2":string, "Sunshade Number 1":string, "Keyence tuning bank idx":i32}, "AP Test Data":cluster{"Raw Sunshade AP Data":string, "Raw Glass AP Data":string, "PMAC Read Counter":dbl, "Database AP Data":dbl[]}, "Motion Status":cluster{"hmi operator abort start time":u32, "Current Data Index":i32, "Analog Data":sgl[][], "Motor Position Hex":u16, "Messages Index":u16, "Last Bytes":u8[], "Current Hall Position":i16, "Motion Stop Timer":u32, "Position Test":T21, "Noise Test":T21, "motion stop check initialized":bool, "remote sense enabled":bool, "Motion":T3}, "LVDT Status":cluster{"LVDT's stored config":T22[], "lvdt precision":T23}, "Sequence State":T24, "misc status":cluster{"delay start time (ticks)":u32, "In Vehicle Mode?":bool, "Diag Mode?":bool, "Serial Port Configured?":bool, "PS Voltage":dbl, "Diag Serial Port":refnum<visa-resource-name>, "Part Setup":T26, "Part History Number":string, "Plant Number":u8, "AP Data Type":T13, "Real Rollo?":bool}, "NVH Operator?":bool, "NVH Pass?":bool, "Operator Pass?":bool, "Operator Action?":bool, "Noise Source":u32, "USBHandle":i32, "PeakInfo":string, "PeakNumber":i32, "NVH Motion Steps":string[], "Second Check?":bool, "Decibel data":dbl[], "Direct Control Info":cluster{"EnableStopOnHome":bool, "EnableStopOnPos":bool, "TeachEvent":bool, "open offset":i32, "close offset":i32, "Derect control":bool, "set position":i32[], "teach pass ":bool, "Drift offsets":i32[], "Hall Positions":i32[]}, "manual control(direct)":bool, "LIN INFO":T31, "Config Info":T34}
  T2 = typedef "All Switch Configuration Cluster.ctl" = cluster{"All Motions":T3, "A":bool[], "B":bool[], "C":bool[], "D":bool[], "A activation time (ms)":u32, "B activation time (ms)":u32, "C activation time (ms)":u32}
  T3 = typedef "All Motions.ctl" = enum16{"Glass Teach", "Glass Slide Open", "Glass Slide Close", "Glass Vent Open", "Glass Vent Close", "Sunshade Teach", "Sunshade Open", "Sunshade Close", "Idle", "Sunshade Open 2", "Sunshade Close 2", "Glass Slide Open Sunshade Open", "Glass Slide Open Sunshade Close", "Glass Slide Close Sunshade Open", "Glass Slide Close Sunshade Close", "Glass Vent Open Sunshade Open", "Glass Vent Open Sunshade Close", "Glass Vent Close Sunshade Open", "Glass Vent Close Sunshade Close", "Express Glass Slide Open", "Express Glass Slide Close", "Express Glass Vent Open", "Express Glass Vent Close", "Express Sunshade Open", "Express Sunshade Close", "Express Sunshade Open 2", "Express Sunshade Close 2", "Express Glass Slide Open Sunshade Open", "Express Glass Slide Open Sunshade Close", "Express Glass Slide Close Sunshade Open", "Express Glass Slide Close Sunshade Close", "Express Glass Vent Open Sunshade Open", "Express Glass Vent Open Sunshade Close", "Express Glass Vent Close Sunshade Open", "Express Glass Vent Close Sunshade Close", "Goto Position Glass", "Goto Position Sunshade", "Sunshade Teach 2"}
  T4 = typedef "EOL Switch Value Configuration Cluster.ctl" = cluster{"All Motions":T3, "Array":T5[]}
  T5 = typedef "EOL Switch Max Min Check Cluster.ctl" = cluster{"Min":dbl, "Max":dbl, "Check?":bool}
  T6 = typedef "station nvh config.ctl" = cluster{"NVH Station?":bool, "nvh app instance path":string, "NVH_ErrorMessages sv url":string, "NVH_Inputs sv url":string, "NVH_MotionNumber sv url":string, "NVH_Outputs sv url":string, "NVH_PartNumber sv url":string, "NVH_PartNumber_Echo sv url":string, "NVH_SerialNumber sv url":string, "NVH_AmbientTempF sv url":string}
  T7 = typedef "station rs232 port map.ctl" = cluster{"PMAC":refnum<visa-resource-name>, "PS Port":refnum<visa-resource-name>, "LVDT Unit":refnum<visa-resource-name>, "RS232":refnum<visa-resource-name>}
  T8 = typedef "station ethernet address map.ctl" = cluster{"LVDT 1 Unit":string, "LVDT Unit 1 port":u16}
  T9 = typedef "station paths.ctl" = cluster{"Base Path":path, "system error log path":path, "Error Table Path":path, "Store errors log path":path, "data bytes log path":path, "network path":path}
  T10 = typedef "EOL Save Module Test Data Control.ctl" = cluster{"Motion Data Array":T11[], "Error Table":string[][], "Sun Shade Close Force Limits":T14, "Sun Shade Open Force Limits":T14, "Sunshade Open Data":sgl[], "Sunshade Close Data":sgl[], "Module Info":T15, "Sunsahde Close Raw Data":sgl[], "Sunshade Open Raw Data":sgl[], "Software Version":string[], "Constant Version":string[], "Hardware Version":string[], "Inalfa Part Number ECU":string[], "LVDT Data":sgl[], "Communication Line 1":sgl[], "Communication Line 2":sgl[], "Anti Pinch Force":sgl[], "Cycle Time":string, "Anti Pinch Vent Force":sgl[], "iGPS LVDT Data":sgl[], "data bytes log":string}
  T11 = typedef "EOL Motion Database Table.ctl" = cluster{"Motion":T3, "Actual Avg Current":dbl, "Actual Runtime":dbl, "Actual Speed":dbl, "Current Data":sgl[], "Motion Data Limits":T12, "Switch 1 to 6":dbl[], "Actual PS Voltage":dbl, "AP Data":i16[][], "Actual max Current":dbl, "Actual Noise (dB)":dbl}
  T12 = typedef "17x Audit Motion Data Seq Control.ctl" = cluster{"Power Supply Voltage":dbl, "Min Avg Current":dbl, "Max Avg Current":dbl, "Min Run Time":dbl, "Max Run Time":dbl, "Min Speed":dbl, "Max Speed":dbl, "AP Data % of Threshold":dbl, "Travel Distance":dbl, "AP Data Type":T13, "Check Current":bool, "Check Run Time":bool, "Check Speed":bool, "Express Motion?":bool, "Check Sound Test":bool, "Check Position?":bool, "Collect AP Data":bool, "Inital Position":u16, "End Position":u16, "Goto Posiition":u16, "Max max Current":dbl, "Min max Current":dbl, "Check max Current":bool, "Check Sound":bool, "Min Sound (dB)":dbl, "Max Sound (dB)":dbl, "SW Mode":enum16{"Hard Switch", "Uncond Frame"}, "LIN Msg":cluster{"ID":u8, "Msg":u8[][], "LDF":refnum<k21>}}
  T13 = typedef "17x AP Data Type.ctl" = enum16{"91/61", "92/62", "93/63", "67", "68", "6F", "71", "91 Msg", "92 Msg", "93 Msg", "94 Msg", "HiRain 91", "HiRain 92 Speed", "HiRain 92 HS", "HiRain 92", "HiRain 93", "SnT"}
  T14 = typedef "17x Sunshade Limts Seq.ctl" = cluster{"Overall Min":dbl, "Overall Max":dbl, "Avg Min":dbl, "Avg Max":dbl, "Truncation Start":dbl, "Truncation End":dbl, "Variance":dbl, "Check Noise":bool}
  T15 = typedef "EOL Module Info Control.ctl" = cluster{"Serial Number":string, "Pallet Number":string, "Sunshade Color":string, "Inalfa Part Number":string, "Customer Number":string}
  T16 = typedef "station DI map.ctl" = cluster{"Abort Test":T17, "Start Test":T17}
  T17 = typedef "EOL Global Digital Input Control.ctl" = enum16{"Dev2/port0/line0", "Dev2/port0/line1", "Dev2/port0/line2", "Dev2/port0/line3", "Dev2/port0/line4", "Dev2/port0/line5", "Dev2/port0/line6", "Dev2/port0/line7", "Dev2/port1/line0", "Dev2/port1/line1", "Dev2/port1/line2", "Dev2/port1/line3", "Dev2/port1/line4", "Dev2/port1/line5", "Dev2/port1/line6", "Dev2/port1/line7", "Dev2/port2/line0", "Dev2/port2/line1", "Dev2/port2/line2", "Dev2/port2/line3", "Dev2/port2/line4", "Dev2/port2/line5", "Dev2/port2/line6", "Dev2/port2/line7", "Prerun Start Test", "Prerun Abort Test", "Audit Start Test", "Audit Abort Test", "Dev2/port3/line4", "Dev2/port3/line5", "Breakin Start Test", "Breakin Abort Test", "Not Implemented"}
  T18 = typedef "control refs.ctl" = cluster{"Start Test":refnum<vi>, "Abort Test":refnum<vi>, "Manual Control":refnum<vi>, "Route to Repair":refnum<vi>, "Waveform Graph":refnum<vi>, "Motion Data":refnum<vi>, "all station status":refnum<vi>, "Individual Station Status":refnum<vi>, "exit program":refnum<vi>, "Sunshade Servo Data Open":refnum<vi>, "Sunshade Servo Data Close":refnum<vi>, "Red-Rabbit Mode":refnum<vi>, "Direct Manual Ctrl":refnum<vi>}
  T19 = typedef "misc station config.ctl" = cluster{"Station Name":string, "is AT station?":bool, "is audit station?":bool, "power supply type":T20, "use alt China TP2 LVDT Logic Seq":bool, "hmi operator abort timeout":u32, "dump all analog values even if pass":bool, "debug log pre-filter ap stream bytes":bool, "use separate lvdt x and z extend tags":bool, "is print":bool}
  T20 = typedef "power supply types.ctl" = enum16{"GENser", "ZUPser", "GENeth", "Manual", "ITECH"}
  T21 = typedef "Pass Fail Control.ctl" = enum16{"Not Tested", "Pass", "Fail"}
  T22 = typedef "EOL LVDT's Check Controller.ctl" = cluster{"Upper Limit":dbl, "Lower Limit":dbl, "LVDT Name":string, "Check":bool}
  T23 = typedef "lvdt precision.ctl" = cluster{"truncate instead of rounding":bool, "decimal places":u8}
  T24 = typedef "sequence state.ctl" = cluster{"Step Description":string, "Cycle Start Time":u32, "Step Data String":string, "Pass?":bool, "Seqence":T25[], "Active Step":u8, "Testing?":bool, "Red-Rabbit Mode":bool, "route-to-repair mode":bool, "NVH Status":cluster{"Restart IRQ Counter":u8, "NVH Test Needed?":bool, "NVH Test Running?":bool}, "Present (s)":dbl, "Hold Mode?":bool, "Hold?":bool, "Rx Invalid?":bool}
  T25 = typedef "Sequence Info.ctl" = cluster{"Name":string, "Description":string, "data string":string}
  T26 = typedef "EOL Part Setup.ctl" = cluster{"Communication Type":T27, "Send Messages to":T28, "RAP Signal":T29, "Motor Type":T30, "NVH Part Number":u16, "Turn Off Timer":u16, "Part Type":string}
  T27 = typedef "All Communication Types.ctl" = enum16{"None", "CAN", "RS 232", "RS 232 LIN", "GM LIN", "SnT LIN", "K Line", "Robel CAN", "P42M-Continental", "Inalfa SCU LIN", "Spare 3"}
  T28 = typedef "Communication with Motors.ctl" = enum16{"Glass", "Rollo", "Both"}
  T29 = typedef "RAP Signal Control.ctl" = enum16{"High", "Low", "None"}
  T30 = typedef "EOL Motor Type.ctl" = enum16{"Smart Motor", "Sensor Motor"}
  T31 = typedef "station LIN config.ctl" = cluster{"Toolkit Type":enum16{"Inalfa LIN", "ADCS LIN", "TS LIN"}, "NAD":u8, "Inalfa LIN":T32, "ADCS LIN":T33, "TS LIN":cluster{"ref info":refnum<k24>, "LIN Channel":i32, "ByteCmd Path":path}}
  T32 = typedef "LIN Device.ctl" = cluster{"Master Frame(3C)":refnum<k21>, "Slave Frame(3D)":refnum<k21>, "Request Schedule":refnum<k21>, "Response Schedule":refnum<k21>, "Frame Write SCU":refnum<k21>, "Frame Read SCU":refnum<k21>, "LIN Name":refnum<k21>}
  T33 = typedef "ADCS_LIN info.ctl" = cluster{"Port":string, "HW select":u16, "XNET Cluster":string, "ByteCmd Path":path}
  T34 = typedef "Config Info.ctl" = variant
  T35 = enum32{"Analog and Digital IO", "Communications", "RSLinx Tags Read", "RSLinx Tags Write", "Barcode Read and Print", "LVDT's", "IO Map", "PMAC Data"}
  T36 = typedef "debug io digital io.ctl" = cluster{"channel name":string, "state":bool}
  T37 = typedef "EOL Analog Input Control.ctl" = enum16{"SW PS  Volage", "Switch A", "Switch B", "Switch C", "Motor Voltage", "Motor Current", "ATS"}
  T38 = typedef "LIN sequence for self SCU.ctl" = string
  T39 = enum32{"Blank", "Cycles", "Read Cycles", "Software Level", "Hardware Level", "Calfile Level", "Tx", "Tx and Rx", "Go to position", "Check positions", "BYD Teach"}
  T40 = cluster{"Step Description":string, "Cycle Start Time":u32, "Step Data String":string, "Pass?":bool, "Seqence":cluster{"Name":string, "Description":string, "data string":string}[], "Active Step":u8, "Testing?":bool, "Red-Rabbit Mode":bool, "route-to-repair mode":bool, "NVH Status":cluster{"Restart IRQ Counter":u8, "NVH Test Needed?":bool, "NVH Test Running?":bool}, "Present (s)":dbl, "Hold Mode?":bool, "Hold?":bool, "Rx Invalid?":bool}
  T41 = cluster{"Sequence State in":cluster{"Step Description":string, "Cycle Start Time":u32, "Step Data String":string, "Pass?":bool, "Seqence":cluster{"Name":string, "Description":string, "data string":string}[], "Active Step":u8, "Testing?":bool, "Red-Rabbit Mode":bool, "route-to-repair mode":bool, "NVH Status":cluster{"Restart IRQ Counter":u8, "NVH Test Needed?":bool, "NVH Test Running?":bool}, "Present (s)":dbl, "Hold Mode?":bool, "Hold?":bool, "Rx Invalid?":bool}, "millisecond timer value":u32, "LVDT's Data Array":T22[], "error out":errorcluster}
  T42 = typedef "EOL Global Digital Output Cluster Control.ctl" = cluster{"Status":bool, "Global DO Ch":T43}
  T43 = typedef "EOL Global Digital Output Control.ctl" = enum16{"Battery", "IGN High", "IGN Low", "LIN", "CAN", "Switch 1", "Switch 2", "Switch 3", "Switch 4", "Switch 5", "Switch 6", "Glass Analog Switch 1", "Glass Analog Switch 2", "Glass Analog Switch 3", "Glass Analog Switch 4", "Sunshade Analog Switch 1", "Sunshade Analog Switch 2", "Sunshade Analog Switch 3", "Sunshade Analog Switch 4", "Glass Motor Relay 1", "Glass Motor Relay 2", "Sunshade Motor Relay 1", "Sunshade Motor Relay 2"}
  T44 = enum16{"Init", "Write", "Write All", "Clear All", "Stop"}
  T45 = typedef "barcode format params.ctl" = cluster{"Format String":string, "Print String":string, "Quantity":u8, "printer type":T46, "RS232 Port":string, "IP Address":string, "Ethernet Port":u32}
  T46 = typedef "barcode printer types.ctl" = enum16{"Intermec RS232", "Intermec Ethernet"}
  T47 = typedef "LIN show messages.ctl" = cluster{"Slide Cycles":u16, "Vent Cycles":u16, "String":string, "Tx Bytes":u8[][], "Rx Bytes":u8[], "Only Tx1 Bytes":u8[][], "Go to Position":u16, "Check Glass Position":u16, "Checkgalss":bool, "Check Sunshade Position":u16, "Checksunshade":bool}
  T48 = typedef "ByteCmd.ctl" = cluster{"CMD":string, "Byte":string}
  T49 = typedef "plc comms params.ctl" = cluster{"PLC boolean read Tags":T50, "PLC bool write Tags":T53, "PLC string read Tags":T54, "PLC string write Tags":T55, "use opc":bool, "PLC/OPC Path":string}
  T50 = typedef "station plc read boolean tags.ctl" = cluster{"AT glass position":T51, "AT shade position":T51, "AT in glass wand lower pos":T51, "AT in glass wand up pos":T51, "AT in sunshad wand lower pos":T51, "AT in sunshad wand up pos":T51, "AT in wand home pos":T51, "LVDT's Extended":T51, "bolt check 1":T51, "bolt check 2":T51, "bolt check 3":T51, "bolt check 4":T51, "bolt check 5":T51, "bolt check 6":T51, "bolt check 7":T51, "bolt check 8":T51, "start":T51, "abort":T51, "LVDT's Retracted":T51, "manual barcode print":T51, "ss servo at open":T51, "ss servo at close":T51, "ss servo opening":T51, "ss servo closing":T51, "control slide at home":T51, "control slide left good":T51, "control slide left over stroke":T51, "control slide right good":T51, "control slide right over stroke":T51, "wind deflector high speed pos":T51, "wind deflector low speed pos":T51, "AT VentPMACatHome":T51, "AT VentPMACisExtend":T51, "SS Barcode Scanner Bypassed":T51, "Check Frame Barcode":T51, "Z LVDTs Extended":T51, "NVH Operator Pass":T51, "NVH Operator Fail":T51, "NVH Operator Express Glass Open":T51, "NVH Operator Express Glass Close":T51, "NVH Operator Express Rollo Open01":T51, "NVH Operator Express Rollo Close01":T51, "NVH Operator Express Rollo Open02":T51, "NVH Operator Express Rollo Close02":T51, "NVH Operator Vent Open Noise":T51, "NVH Operator Vent Close Noise":T51, "NVH Operator Sunshade Open Noise":T51, "NVH Operator Sunshade Close Noise":T51, "NVH Operator Glass Open Noise":T51, "NVH Operator Glass Close Noise":T51, "NVH Operator Finish":T51, "NVH Operator Check":T51, "windproof position":T51, "NVH Operator Express Glass vent Open":T51, "NVH Operator Express Glass Vent Close":T51, "NVH Operator Re-do":T51, "AT at vent ATS test pos":T51, "AT at vent ATS Home pos":T51, "Start Adjust LVDT":T51, "Finish Adjust LVDT":T51}
  T51 = typedef "plc path and tag.ctl" = cluster{"Tag Name":string, "Network Path":string, "use opc":bool, "DataSocket Reference":T52}
  T52 = typedef "DataSocket Reference Type.ctl" = cluster{"CWDSLib._DCWDataSocket":refnum<k7>, "CWDSLib._DCWData":refnum<k7>, "OnDataUpdated":u32, "OnStatusUpdated":u32}
  T53 = typedef "station plc write boolean tags.ctl" = cluster{"AT set glass wand lower":T51, "AT set sunshade wand lower":T51, "AT set sunshade wand up":T51, "AT set glass wand up":T51, "AT set wand home pos":T51, "Test Complete Pass":T51, "Test Complete Fail":T51, "Test Started":T51, "Retract LVDT's":T51, "Extend LVDT's":T51, "ss servo open":T51, "ss servo close":T51, "control slide start":T51, "control slide stop":T51, "AT VentPMACHome":T51, "AT VentPMACExtended":T51, "Good Frame Barcode":T51, "Bad Frame Barcode":T51, "Extend Z LVDTS":T51, "NVH SunRoof Moving":T51, "NVH SunRoof Stop":T51, "NVH Pass":T51, "NVH Fail":T51, "NVH Operator Express Glass Opened":T51, "NVH Operator Express Glass Closed":T51, "NVH Operator Express Rollo Opened01":T51, "NVH Operator Express Rollo Closed01":T51, "NVH Operator Express Rollo Opened02":T51, "NVH Operator Pass":T51, "NVH Operator Fail":T51, "NVH Operator Check":T51, "NVH Operator Vent Open Noise":T51, "NVH Operator Vent Close Noise":T51, "NVH Operator Sunshade Open Noise":T51, "NVH Operator Sunshade Close Noise":T51, "NVH Operator Glass Open Noise":T51, "NVH Operator Glass Close Noise":T51, "NVH Operator Finish":T51, "Barcode01 OK":T51, "Barcode02 OK":T51, "AT set to Vent ATS Test Pos":T51, "AT set to Vent ATS Home Pos":T51, "Move LVDT Adjust Station":T51}
  T54 = typedef "station plc read string tags.ctl" = cluster{"Serial Number":T51, "Pallet Number":T51, "Inalfa Part Number":T51, "Shade Color":T51, "Model Type":T51, "Customer Number":T51, "Part History Number":T51, "Shade 1 Barcode":T51, "Shade 2 Barcode":T51, "Manual Serial Number":T51, "Manual Inalfa Part Number":T51, "Manual Shade Color":T51, "Manual Model Type":T51, "Manual Customer Number":T51, "Manual Part History Number":T51}
  T55 = typedef "station plc write string tags.ctl" = cluster{"barcode station error":T51, "error message 0":T51, "error message 1":T51, "error message 2":T51, "error message 3":T51}
  T56 = typedef "NI_LVConfig.lvlib/Config Data RefNum.ctl" = refnum<k1>
  T57 = cluster{"ref info":refnum<k24>, "LIN Channel":i32, "ByteCmd Path":path}
  T58 = cluster{"SW":string, "HW":string, "Cal":string, "RP RF":u8, "Hall":cluster{"Glass":i16, "Rollo":i16}, "Cycle":cluster{"Slide":u16, "Vent":u16}, "Hold？":bool}
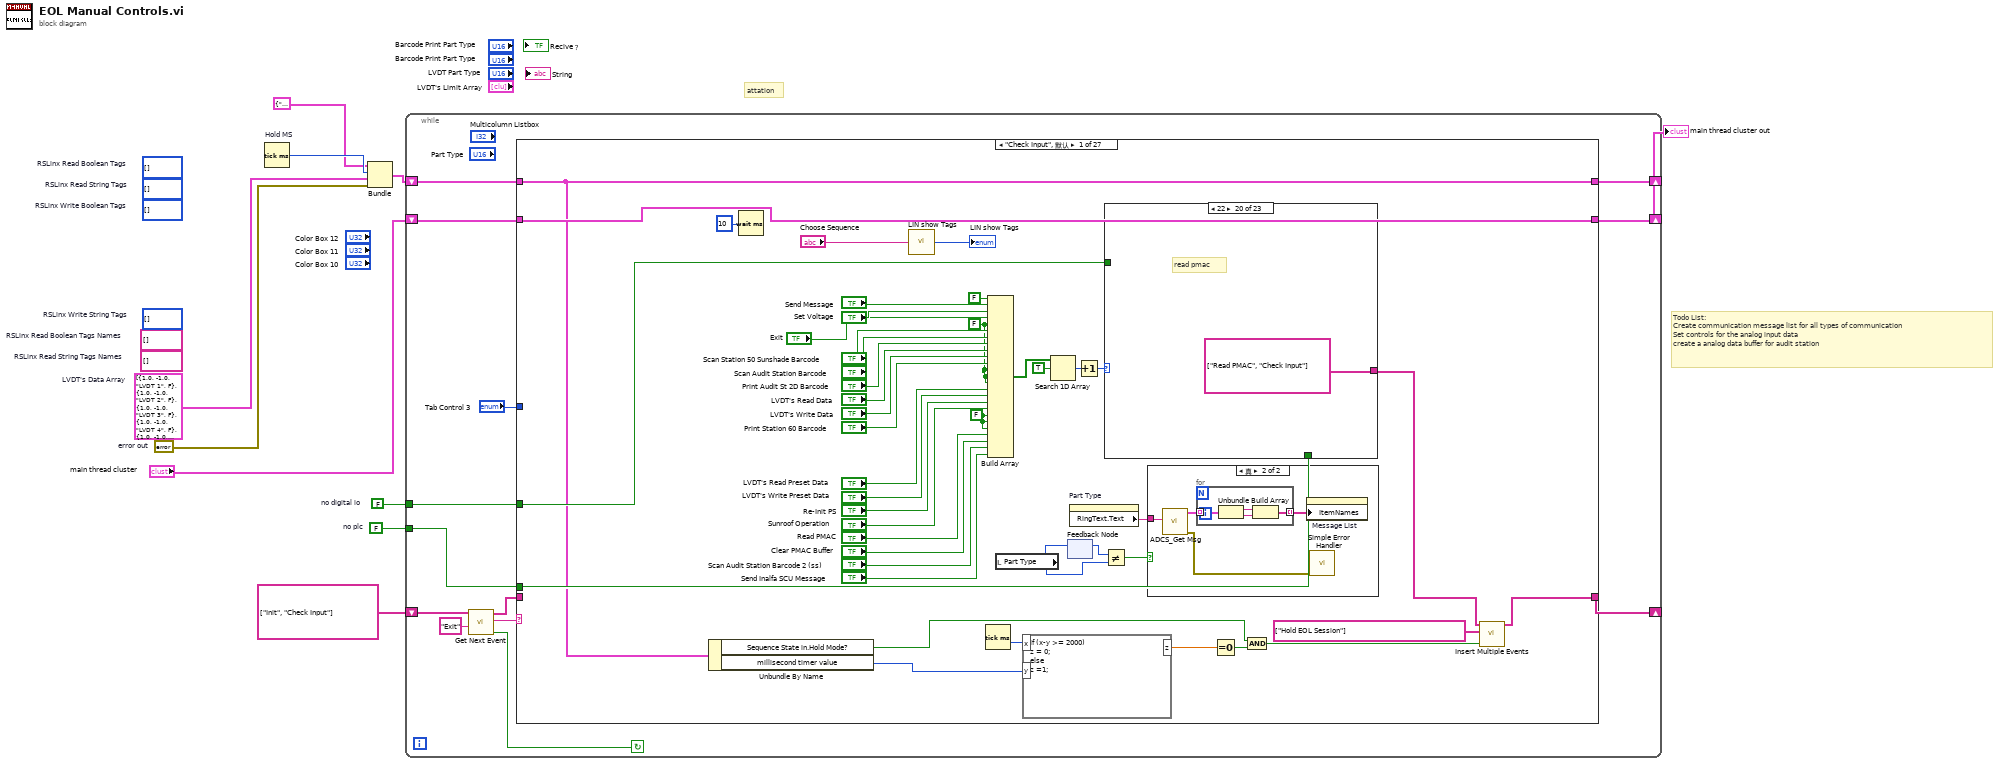
[diagram p0: block diagram]
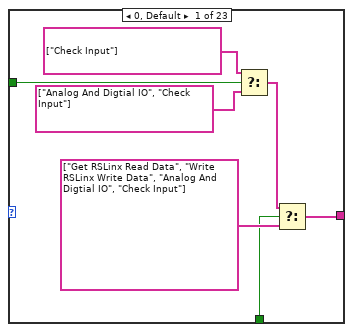
[diagram p3: hidden frame]
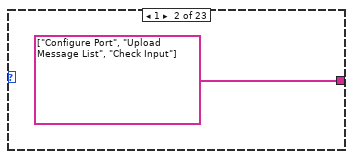
[diagram p4: hidden frame]
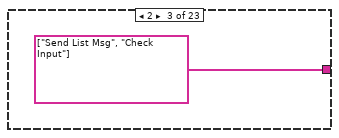
[diagram p5: hidden frame]
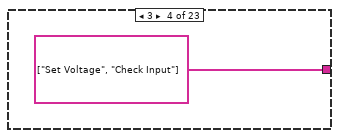
[diagram p6: hidden frame]
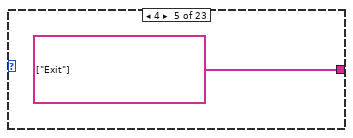
[diagram p7: hidden frame]
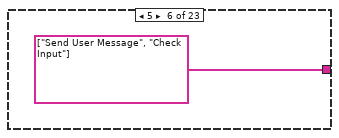
[diagram p8: hidden frame]
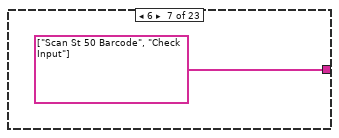
[diagram p9: hidden frame]
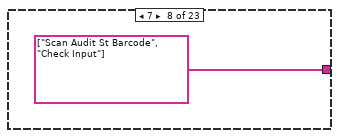
[diagram p10: hidden frame]
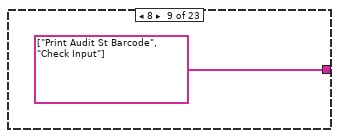
[diagram p11: hidden frame]
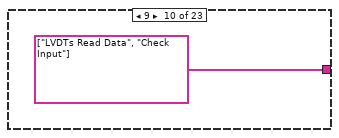
[diagram p12: hidden frame]
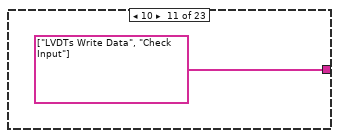
[diagram p13: hidden frame]
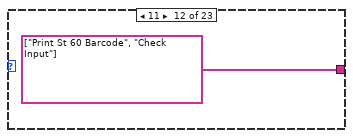
[diagram p14: hidden frame]
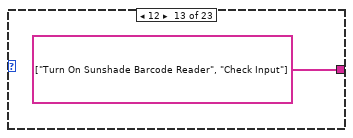
[diagram p15: hidden frame]
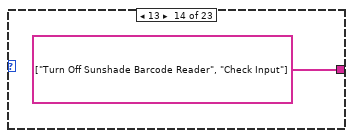
[diagram p16: hidden frame]
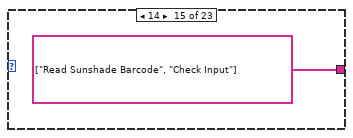
[diagram p17: hidden frame]
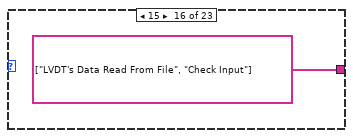
[diagram p18: hidden frame]
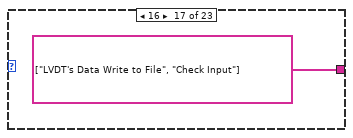
[diagram p19: hidden frame]
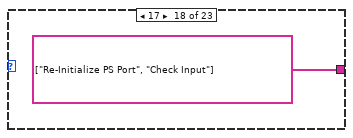
[diagram p20: hidden frame]
diagram:
  w5 = FALSE  # no digital io
  w6 = FALSE  # no plc
  w8 = errorcluster {"status"=FALSE, "code"=0, "source"=""}  # error out
  w9 = T22[] [{"Upper Limit"=1.0, "Lower Limit"=-1.0, "LVDT Name"="LVDT 1", "Check"=FALSE}, {"Upper Limit"=1.0, "Lower Limit"=-1.0, "LVDT Name"="LVDT 2", "Check"=FALSE}, {"Upper Limit"=1.0, "Lower Limit"=-1.0, "LVDT Name"="LVDT 3", "Check"=FALSE}, {"Upper Limit"=1.0, "Lower Limit"=-1.0, "LVDT Name"="LVDT 4", "Check"=FALSE}, {"Upper Limit"=1.0, "Lower Limit"=-1.0, "LVDT Name"="LVDT 5", "Check"=FALSE}, {"Upper Limit"=1.0, "Lower Limit"=-1.0, "LVDT Name"="LVDT 6", "Check"=FALSE}, {"Upper Limit"=1.0, "Lower Limit"=-1.0, "LVDT Name"="LVDT 7", "Check"=FALSE}, {"Upper Limit"=1.0, "Lower Limit"=-1.0, "LVDT Name"="LVDT 8", "Check"=FALSE}, {"Upper Limit"=1.0, "Lower Limit"=-1.0, "LVDT Name"="LVDT 9", "Check"=FALSE}, {"Upper Limit"=1.0, "Lower Limit"=-1.0, "LVDT Name"="LVDT 10", "Check"=FALSE}, {"Upper Limit"=1.0, "Lower Limit"=-1.0, "LVDT Name"="LVDT 11", "Check"=FALSE}, {"Upper Limit"=1.0, "Lower Limit"=-1.0, "LVDT Name"="LVDT 12", "Check"=FALSE}, {"Upper Limit"=1.0, "Lower Limit"=-1.0, "LVDT Name"="LVDT 13", "Check"=FALSE}, {"Upper Limit"=1.0, "Lower Limit"=-1.0, "LVDT Name"="LVDT 14", "Check"=FALSE}]  # LVDT's Data Array
  (unwired) string[] []  # RSLinx Read String Tags Names
  (unwired) string[] []  # RSLinx Read Boolean Tags Names
  (unwired) i32[] []  # RSLinx Write String Tags
  (unwired) i32[] []  # RSLinx Write Boolean Tags
  (unwired) i32[] []  # RSLinx Read String Tags
  (unwired) i32[] []  # RSLinx Read Boolean Tags
  # "attation"
  # "Todo List:\nCreate communication message list for all types of communication \nSet controls for the analog input data\ncreate a analog data buffer for audit station"
  n1 = Tick Count (ms) "Hold MS"() -> (millisecond timer value=w2:u32)
  n2 = Bundle("Sequence State in"=T40 {"Step Description"="", "Cycle Start Time"=0, "Step Data String"="", "Pass?"=FALSE, "Seqence"=[], "Active Step"=0, "Testing?"=FALSE, "Red-Rabbit Mode"=FALSE, "route-to-repair mode"=FALSE, "NVH Status"={"Restart IRQ Counter"=0, "NVH Test Needed?"=FALSE, "NVH Test Running?"=FALSE}, "Present (s)"=0.0, "Hold Mode?"=FALSE, "Hold?"=FALSE, "Rx Invalid?"=FALSE}, "millisecond timer value"=w2, "LVDT's Data Array"=w9, "error out"=w8) -> (w10:T41)  [unwired: 1 in]
  n3 = while {
    shift-right: [w22] -> _
    shift-left: string[] ["Init", "Check Input"] ("event queue out") -> [w14]
    shift-right: [w20] -> _
    shift-left: w10 -> [w21]
    shift-right: [w17] -> w7
    shift-left: "main thread cluster" -> [w13]
    tunnel: w6 -> [w16]
    tunnel: w5 -> [w15]
    stop <- w19 continue-if-true
    n4 = call "Get Next Event.vi"("Exit Event"="Exit", "event queue in"=w14) -> ("Condition (Exit:F)"=w19:bool, "next event"=w23:string, "event queue out"=w12:string[])  [unwired: 3 in]
    n5 = case shown="\"Check Input\", 默认" w23 {
      tunnel: w12 -> [_ w109 w128 w150 w154 w164 w240 w276 w289 w306 w322 w347 w385 w414 w440 w547 w588 w635 w645 w674 w709 w713 _ w722 w734 w745 w763]
      tunnel: [w37 w109 w128 w150 w154 w164 w240 w276 w289 w305 w322 w347 w385 w414 w440 w547 w588 w635 w645 w674 w709 w713 string[] ["Check Input"] ("event queue out") w722 w734 w745 w763] -> w22
      tunnel: w21 -> [w35 w110 w129 w149 w158 w163 w220 w275 w290 w303 w324 w346 w384 w415 w425 w542 w579 w634 w644 w673 w710 w714 w718 w723 w735 w751 w767]
      tunnel: [w35 w110 w129 w149 w158 w163 w220 w275 w290 w303 w324 w346 w384 w412 w424 w546 w578 w634 w644 w673 w710 w714 w718 w723 w735 w751 w767] -> w20
      tunnel: w13 -> [w49 w106 w115 w148 w155 w160 w215 w263 w278 w302 w321 w342 w381 w410 w431 w553 w593 w633 w641 w670 w712 w715 w717 w720 w732 w746 w764]
      tunnel: [w49 w106 w115 w148 w156 w160 w215 w263 w278 w302 w321 w342 w381 w410 w431 w553 w593 w633 w641 w670 w712 w715 w717 w720 w732 w746 w764] -> w17
      tunnel: w16 -> [w48 _ _ _ _ _ _ _ _ _ _ _ _ _ _ _ _ _ _ _ _ _ _ _ _ _ _]
      tunnel: w15 -> [w47 _ _ _ _ _ _ _ _ _ _ _ _ _ _ _ _ _ _ _ _ _ _ w721 w733 _ _]
      tunnel: "Tab Control 3" -> [_ _ _ _ _ w162 _ _ _ _ _ _ _ _ _ _ _ _ _ w672 _ _ _ _ _ _ _]
      frame "Check Input", Default {
        w24 = FALSE ("元素")
        w40 = FALSE ("元素")
        n6 = Unbundle By Name(w35) -> ("Sequence State in.Hold Mode?"=w31:bool, "millisecond timer value"=w33:u32)
        n7 = Wait (ms)(milliseconds to wait=u32 10) -> ()  [unwired: 1 out]
        n8 = call "LIN show Tags.vi"("Choose Sequence"="Choose Sequence") -> ("LIN show Tags"=→"LIN show Tags":T39)  [unwired: 4 in]
        n9 = Tick Count (ms)() -> (millisecond timer value=w34:u32)
        n10 = Build Array(FALSE ("元素"), "Send Message", "Set Voltage", "Exit", w24, "Scan Station 50 Sunshade Barcode", "Scan Audit Station Barcode", "Print Audit St 2D Barcode", "LVDT's Read Data", "LVDT's Write Data", "Print Station 60 Barcode", w24, w24, w24, "LVDT's Read Preset Data", "LVDT's Write Preset Data", "Re-Init PS", "Sunroof Operation", w40, w40, w40, "Read PMAC", "Clear PMAC Buffer", "Scan Audit Station Barcode 2 (ss)", "Send Inalfa SCU Message") -> (w64:bool[])
        n11 = local read "Part Type"() -> (w27:u16)
        n12 = formula code="if (x-y >= 2000) \nz = 0;\nelse\nz =1;"("x"=w34, "y"=w33) -> ("z"=w32:dbl)
        n13 = Search 1D Array(1D array=w64, element=TRUE) -> (index of element=w62:i32)  [unwired: 1 in]
        n14 = feedback #1() -> (w28:u16)  [unwired: 1 in]
        n15 = feedback-in #1(w27) -> ()
        n16 = property on="Part Type" class="Ring (严格)"() -> ("RingText.Text"=w25:string)  [unwired: 2 in, 2 out]
        n17 = Increment(x=w62) -> (x+1=w61:i32)
        n18 = Not Equal?(x=w28, y=w27) -> (x != y?=w26:bool)
        n19 = case shown="22" w61 {
          tunnel: [w80 string[] ["Configure Port", "Upload Message List", "Check Input"] ("event queue out") string[] ["Send List Msg", "Check Input"] ("event queue out") string[] ["Set Voltage", "Check Input"] ("event queue out") string[] ["Exit"] ("event queue out") string[] ["Send User Message", "Check Input"] ("event queue out") string[] ["Scan St 50 Barcode", "Check Input"] ("event queue out") string[] ["Scan Audit St Barcode", "Check Input"] ("event queue out") string[] ["Print Audit St Barcode", "Check Input"] ("event queue out") string[] ["LVDTs Read Data", "Check Input"] ("event queue out") string[] ["LVDTs Write Data", "Check Input"] ("event queue out") string[] ["Print St 60 Barcode", "Check Input"] ("event queue out") string[] ["Turn On Sunshade Barcode Reader", "Check Input"] ("event queue out") string[] ["Turn Off Sunshade Barcode Reader", "Check Input"] ("event queue out") string[] ["Read Sunshade Barcode", "Check Input"] ("event queue out") string[] ["LVDT's Data Read From File", "Check Input"] ("event queue out") string[] ["LVDT's Data Write to File", "Check Input"] ("event queue out") string[] ["Re-Initialize PS Port", "Check Input"] ("event queue out") string[] ["Sunroof Operation", "Check Input"] ("event queue out") string[] ["Read PMAC", "Check Input"] ("event queue out") string[] ["Clear PMAC Buffer", "Check Input"] ("event queue out") string[] ["Scan Audit St Barcode 2", "Check Input"] ("event queue out") string[] ["Send Inalfa SCU Message", "Check Input"] ("event queue out")] -> w38
          tunnel: w48 -> [w81 _ _ _ _ _ _ _ _ _ _ _ _ _ _ _ _ _ _ _ _ _ _]
          tunnel: w47 -> [w77 _ _ _ _ _ _ _ _ _ _ _ _ _ _ _ _ _ _ _ _ _ _]
          frame 0, Default {
            n20 = Select(t=string[] ["Check Input"] ("event queue out"), s=w77, f=string[] ["Analog And Digtial IO", "Check Input"] ("event queue out")) -> (s? t:f=w78:string[])
            n21 = Select(t=w78, s=w81, f=string[] ["Get RSLinx Read Data", "Write RSLinx Write Data", "Analog And Digtial IO", "Check Input"] ("event queue out")) -> (s? t:f=w80:string[])
          }
          frame 1 {
          }
          frame 2 {
          }
          frame 3 {
          }
          frame 4 {
          }
          frame 5 {
          }
          frame 6 {
          }
          frame 7 {
          }
          frame 8 {
          }
          frame 9 {
          }
          frame 10 {
          }
          frame 11 {
          }
          frame 12 {
          }
          frame 13 {
          }
          frame 14 {
          }
          frame 15 {
          }
          frame 16 {
          }
          frame 17 {
          }
          frame 18 {
          }
          frame 22 {
            # "read pmac"
          }
          frame 23 {
            # "clear pmac buffers"
          }
          frame 24 {
          }
          frame 25 {
          }
        }
        n22 = case shown="真" w26 {
          tunnel: w25 -> [_ w71]
          frame False {
          }
          frame True {
            n23 = call <vilib>:"ADCS_Get Msg.vi"("Mode type"=w71) -> ("错误输出"=w68:errorcluster, "LIN Msg"=w70:T48[])  [unwired: 6 in, 2 out]
            n24 = for {
              tunnel: w70 -> [w75] mode=indexing
              tunnel: [w72] -> w69 mode=indexing
              n25 = Unbundle(w75) -> ("CMD"=w74:string, "Byte"=w73:string)
              n26 = Build Array(w74, w73) -> (w72:string[])
            }
            n27 = property on="Message List" class="MCListbox (严格)"("ItemNames"=w69) -> ()  [unwired: 2 in, 2 out]
            n28 = call <vilib>:"Simple Error Handler.vi"("error in (no error)"=w68) -> ()  [unwired: 4 in, 5 out]
          }
        }
        n29 = Equal To 0?(x=w32) -> (x = 0?=w30:bool)
        n30 = And(x=w31, y=w30) -> (x .and. y?=w29:bool)
        n31 = call "Insert Multiple Events.vi"("Insert all? (T)"=w29, "Events to Insert"=string[] ["Hold EOL Session"], "Event queue in"=w38) -> ("Event queue out"=w37:string[])  [unwired: 4 in]
      }
      frame "Sunroof Operation" {
        n32 = Unbundle By Name(w106) -> ("misc station config.Station Name"=w107:string, "Station Index"=w108:i32)
        n33 = Unbundle By Name(w106) -> ("DO Task"=w105:refnum<k21>)
        n34 = call "EOL Manual Sunroof Control.vi"("DO Task"=w105, "station name"=w107, "station idx"=w108) -> ()  [unwired: 9 in]
      }
      frame "Analog And Digtial IO" {
        n35 = Unbundle By Name(w115) -> ("Station Index"=w125:i32, "D in map"=w123:T16)
        n36 = Unbundle By Name(w115) -> ("DO Task"=w114:refnum<k21>)
        n37 = call "EOL All-Station AI Circular Data Buffer.vi"("station idx"=w125, "Mode"=enum16{"Initialize", "Read", "Write"}."Read") -> ("Data Read (Samp-Ro, Ch-Col)"=w126:sgl[][])  [unwired: 9 in]
        n38 = Cluster To Array(cluster=w123) -> (array=w120:T17[])
        n39 = for {
          tunnel: "Digital Output Array" -> [w147] mode=indexing
          tunnel: [w145] -> w112 mode=indexing
          tunnel: T42 {"Status"=FALSE, "Global DO Ch"=enum."Battery"} ("Cluster") -> [w144]
          n40 = Unbundle By Name(w147) -> ("channel name"=w142:string, "state"=w146:bool)
          n41 = Scan From String(input string=w142, default 1=EOL_Global_Digital_Output_Control."Battery" ("Global DO Ch")) -> (output 1=w141:T43)  [unwired: 3 in, 3 out]
          n42 = Bundle By Name(cluster=w144, "Global DO Ch"=w141, "Status"=w146) -> (w145:T42)
        }
        n43 = Index Array(array=w126, index (col) #1="Analog Control", index (col) #2="Analog Control 2", index (col) #3="Analog Control 3") -> (element #1=w130:sgl[], element #2=w131:sgl[], element #3=w132:sgl[])  [unwired: 3 in]
        n44 = Build Array(w130, w131, w132) -> (→"Audit Graph":sgl[][])
        n45 = local read "All Inputs"() -> (w122:T36[])
        n46 = call "EOL Digital Inputs v2.vi"("Digital Inputs Array"=w120, "Mode"=enum16{"Init", "Read", "Read All", "Close"}."Read") -> ("DI Status"=w121:bool[])  [unwired: 7 in, 2 out]
        n47 = Empty Array?(array=w112) -> (empty?=w111:bool)
        n48 = case shown="假" w111 {
          tunnel: w114 -> [w136 _]
          tunnel: w112 -> [w135 _]
          frame False {
            n49 = call "EOL Digital Outputs v3.vi"("task/channels in"=w136, "DO Status"=w135, "Mode"=T44."Write") -> ()  [unwired: 7 in, 2 out]
          }
          frame True {
          }
        }
        n50 = for {
          tunnel: w122 -> [w140] mode=indexing
          tunnel: w121 -> [w138] mode=indexing
          tunnel: [w139] -> w119 mode=indexing
          n51 = Bundle By Name(cluster=w140, "state"=w138) -> (w139:T36)
        }
        "All Inputs" <- w119
      }
      frame "Error" {
      }
      frame "Exit" {
        n52 = Unbundle By Name(w155) -> ("misc status.Diag Serial Port"=w157:refnum<visa-resource-name>)  [unwired: 1 out]
        n53 = VISA Close(VISA resource name=w157) -> (error out=w151:errorcluster)  [unwired: 1 in]
        n54 = call <vilib>:"Clear Errors.vi"("error in (no error)"=w151) -> ()  [unwired: 5 in, 2 out]
        n55 = Bundle By Name(cluster=w155, "misc status.Serial Port Configured?"=FALSE ("Serial Port Configured?")) -> (w156:T1)
        n56 = local write "Communications Tab"(enum32{"Send Message"}."Send Message" ("Communications Tab")) -> ()
      }
      frame "Get RSLinx Read Data" {
        n57 = Unbundle By Name(w160) -> ("Config Info"=w161:T34)
        n58 = call "Config Info Get.vi"("Config Info"=w161) -> ("PLC Comms"=w159:T49)  [unwired: 7 in, 3 out]
        n59 = case shown="\"RSLinx Tags Read\"" w162 {
          tunnel: w159 -> [_ w175]
          frame "Analog and Digital IO", Default {
          }
          frame "RSLinx Tags Read" {
            w166 = errorcluster {"status"=FALSE, "code"=0, "source"=""} ("error out")
            n60 = Unbundle By Name(w175) -> ("PLC boolean read Tags"=w170:T50, "PLC string read Tags"=w173:T54)
            n61 = Cluster To Array(cluster=w170) -> (array=w169:T51[])
            n62 = Cluster To Array(cluster=w173) -> (array=w174:T51[])
            n63 = for {
              tunnel: w169 -> [w178] mode=indexing
              tunnel: [w181] -> w171 mode=indexing
              shift-right: [w177] -> w168
              shift-left: w166 -> [w176]
              n64 = Unbundle By Name(w178) -> ("Tag Name"=w180:string)
              n65 = Empty String/Path?(string/path=w180) -> (empty?=w179:bool)
              n66 = case shown="假" w179 {
                tunnel: w180 -> [w189 _]
                tunnel: [w188 _] -> w181
                tunnel: w178 -> [w185 _]
                tunnel: [w184 w190] -> w177
                tunnel: w176 -> [w183 w190]
                frame False {
                  n67 = Wait Until Next ms Multiple(millisecond multiple=u32 1) -> ()  [unwired: 1 out]
                  n68 = call "plc read bool.vi"("error in"=w183, "addr,tag"=w185) -> ("error out"=w184:errorcluster, "value"=w186:bool)  [unwired: 8 in]
                  n69 = Bundle By Name(cluster=cluster{"Tag String":string, "Boolean":bool} {"Tag String"="", "Boolean"=FALSE} ("Cluster"), "Tag String"=w189, "Boolean"=w186) -> (w188:cluster{"Tag String":string, "Boolean":bool})
                }
                frame True {
                }
              }
            }
            "RSLinx Read Boolean" <- w171
            n70 = for {
              tunnel: w174 -> [w191] mode=indexing
              tunnel: [w196] -> w172 mode=indexing
              shift-right: [w192] -> w167
              shift-left: w166 -> [w193]
              n71 = Unbundle By Name(w191) -> ("Tag Name"=w194:string)
              n72 = Empty String/Path?(string/path=w194) -> (empty?=w195:bool)
              n73 = case shown="假" w195 {
                tunnel: w194 -> [w202 _]
                tunnel: [w203 _] -> w196
                tunnel: w193 -> [w201 w205]
                tunnel: [w200 w205] -> w192
                tunnel: w191 -> [w198 _]
                frame False {
                  n74 = Wait Until Next ms Multiple(millisecond multiple=u32 1) -> ()  [unwired: 1 out]
                  n75 = call "plc read string.vi"("error in"=w201, "addr,tag"=w198) -> ("error out"=w200:errorcluster, "Data"=w199:string)  [unwired: 8 in]
                  n76 = Bundle By Name(cluster=cluster{"Tag String":string, "String":string} {"Tag String"="", "String"=""} ("Cluster"), "Tag String"=w202, "String"=w199) -> (w203:cluster{"Tag String":string, "String":string})
                }
                frame True {
                }
              }
            }
            "RSLinx Read String" <- w172
            n77 = Merge Errors(w168, w167) -> (→"错误输出":errorcluster)
          }
        }
      }
      frame "Init" {
        w208 = FALSE
        w221 = u16 0
        n78 = Unbundle By Name(w215) -> ("rs232 port map"=→"rs232 port map":T7, "misc station config.Station Name"=w239:string, "LIN INFO.Toolkit Type"=→"Toolkit Type":enum16{"Inalfa LIN", "ADCS LIN", "TS LIN"}, "DO Task"=w207:refnum<k21>)
        n79 = Unbundle By Name(w215) -> ("Config Info"=w216:T34)
        n80 = call "Config Read Part Type.vi"() -> ("Error Out"=w224:errorcluster, "Part Types"=w218:string[])  [unwired: 9 in, 1 out]
        n81 = call "Config Info Get.vi"("Config Info"=w216) -> ("PLC Comms"=w213:T49)  [unwired: 7 in, 3 out]
        n82 = Unbundle By Name(w213) -> ("PLC bool write Tags"=w232:T53, "PLC string write Tags"=w231:T55)
        n83 = property on="Part Type" class="Ring (严格)"("Strings []"=w218) -> ()  [unwired: 2 in, 2 out]
        n84 = property class="DAQmx任务"(reference=w207) -> ("Channels"=w206:refnum<k21>[])  [unwired: 1 in, 2 out]
        n85 = Cluster To Array(cluster=w231) -> (array=w229:T51[])
        n86 = Cluster To Array(cluster=w232) -> (array=w230:T51[])
        n87 = call "enumerate digital io channel names.vi"() -> ("digital inputs"=w235:string[])  [unwired: 10 in, 1 out]
        n88 = for {
          tunnel: cluster{"String":string, "Value":ext} {"String"="", "Value"=0.0} -> [w249]
          tunnel: w218 -> [w247] mode=indexing
          tunnel: [w246] -> w222 mode=indexing
          i -> [w245]
          n89 = To Extended Precision Float(1:w245) -> (0:w248:ext)
          n90 = Bundle By Name(cluster=w249, "String"=w247, "Value"=w248) -> (w246:cluster{"String":string, "Value":ext})
        }
        n91 = for {
          tunnel: w230 -> [w255] mode=indexing
          tunnel: [w254] -> w227 mode=indexing
          tunnel: [FALSE] -> w226 mode=indexing
          n92 = Unbundle By Name(w255) -> ("Tag Name"=w254:string)  [unwired: 1 out]
        }
        "RSLinx Write Tag Boolean Array Names" <- w227
        n93 = for {
          tunnel: w229 -> [w252] mode=indexing
          tunnel: [w251] -> w228 mode=indexing
          tunnel: [""] -> w225 mode=indexing
          n94 = Unbundle By Name(w252) -> ("Tag Name"=w251:string)  [unwired: 1 out]
        }
        "RSLinx Write Tag String Array Names" <- w228
        n95 = for {
          tunnel: w235 -> [w260] mode=indexing
          tunnel: [w259] -> w233 mode=indexing
          n96 = Bundle By Name(cluster=T36 {"channel name"="", "state"=FALSE} ("dio"), "channel name"=w260) -> (w259:T36)
        }
        n97 = for {
          tunnel: w206 -> [w257] mode=indexing
          tunnel: [w256] -> w234 mode=indexing
          n98 = Bundle By Name(cluster=T36 {"channel name"="", "state"=FALSE} ("dio"), "channel name"=w257) -> (w256:T36)
        }
        n99 = Concatenate Strings(w239, " Manual Control" ("string")) -> (→"Title":string)
        n100 = property on="LVDT Part Type" class="Ring (严格)"(error in=w224, "StringsAndValues[]"=w222, "Value"=w221) -> ()  [unwired: 1 in, 2 out]
        n101 = property on="Barcode Print Part Type" class="Ring (严格)"("StringsAndValues[]"=w222, "Value"=w221) -> ()  [unwired: 2 in, 2 out]
        n102 = local write "RSLinx Write Tag Boolean Array Data"(w226) -> ()
        n103 = local write "RSLinx Write Tag String Array Data"(w225) -> ()
        n104 = local write "All Inputs"(w233) -> ()
        n105 = local write "Digital Output Array"(w234) -> ()
        n106 = property on="Barcode Print Part Type" class="Ring (严格)"("StringsAndValues[]"=w222, "Value"=w221) -> ()  [unwired: 2 in, 2 out]
        n107 = property on="Multicolumn Listbox" class="MCListbox (严格)"("ItemNames"=string[][] [] ("项名")) -> ()  [unwired: 2 in, 2 out]
        n108 = property on="Part Type" class="Ring (严格)"() -> ("RingText.Text"=w212:string)  [unwired: 2 in, 2 out]
        n109 = local write "Recive？"(w208) -> ()
        n110 = local write "Hold？"(w208) -> ()
        n111 = call <vilib>:"ADCS_Get Msg.vi"("Mode type"=w212) -> ("错误输出"=w209:errorcluster, "LIN Msg"=w211:T48[])  [unwired: 6 in, 2 out]
        n112 = for {
          tunnel: w211 -> [w244] mode=indexing
          tunnel: [w241] -> w210 mode=indexing
          n113 = Unbundle(w244) -> ("CMD"=w243:string, "Byte"=w242:string)
          n114 = Build Array(w243, w242) -> (w241:string[])
        }
        n115 = call <vilib>:"Simple Error Handler.vi"("error in (no error)"=w209) -> ()  [unwired: 4 in, 5 out]
        n116 = property on="Message List" class="MCListbox (严格)"("ItemNames"=w210) -> ()  [unwired: 2 in, 2 out]
        "Communications Tab" <- enum32{"Send Message"}."Send Message" ("Communications Tab")
      }
      frame "LVDT's Data Read From File" {
        n117 = Unbundle By Name(w263) -> ("paths.Base Path"=w262:path)
        n118 = property on="LVDT Part Type" class="Ring (严格)"() -> ("RingText.Text"=w267:string)  [unwired: 2 in, 2 out]
        n119 = call "get path to lvdt presets.vi"("product"=w267, "paths.Base Path"=w262) -> ("path"=w268:path)  [unwired: 9 in]
        n120 = call <vilib>:"Open Config Data.vi"("configuration file path"=w268) -> ("error out"=w272:errorcluster, "refnum"=w273:T56)  [unwired: 8 in, 1 out]
        n121 = call-poly <vilib>:"Read Key.vi"("section"="LVDT's Preset Data", "error in (no error)"=w272, "key"=w267, "refnum"=w273) -> ("error out"=w266:errorcluster, "value"=w270:string, "refnum out"=w264:T56)  [unwired: 4 in, 1 out]
        n122 = call <vilib>:"Close Config Data.vi"("error in (no error)"=w266, "refnum"=w264) -> ("error out"=w265:errorcluster)  [unwired: 8 in, 1 out]
        n123 = Unflatten From String(type=T22[] [{"Upper Limit"=1.0, "Lower Limit"=-1.0, "LVDT Name"="LVDT 1", "Check"=FALSE}, {"Upper Limit"=1.0, "Lower Limit"=-1.0, "LVDT Name"="LVDT 2", "Check"=FALSE}, {"Upper Limit"=1.0, "Lower Limit"=-1.0, "LVDT Name"="LVDT 3", "Check"=FALSE}, {"Upper Limit"=1.0, "Lower Limit"=-1.0, "LVDT Name"="LVDT 4", "Check"=FALSE}, {"Upper Limit"=1.0, "Lower Limit"=-1.0, "LVDT Name"="LVDT 5", "Check"=FALSE}, {"Upper Limit"=1.0, "Lower Limit"=-1.0, "LVDT Name"="LVDT 6", "Check"=FALSE}, {"Upper Limit"=1.0, "Lower Limit"=-1.0, "LVDT Name"="LVDT 7", "Check"=FALSE}, {"Upper Limit"=1.0, "Lower Limit"=-1.0, "LVDT Name"="LVDT 8", "Check"=FALSE}, {"Upper Limit"=1.0, "Lower Limit"=-1.0, "LVDT Name"="LVDT 9", "Check"=FALSE}, {"Upper Limit"=1.0, "Lower Limit"=-1.0, "LVDT Name"="LVDT 10", "Check"=FALSE}, {"Upper Limit"=1.0, "Lower Limit"=-1.0, "LVDT Name"="LVDT 11", "Check"=FALSE}, {"Upper Limit"=1.0, "Lower Limit"=-1.0, "LVDT Name"="LVDT 12", "Check"=FALSE}, {"Upper Limit"=1.0, "Lower Limit"=-1.0, "LVDT Name"="LVDT 13", "Check"=FALSE}, {"Upper Limit"=1.0, "Lower Limit"=-1.0, "LVDT Name"="LVDT 14", "Check"=FALSE}] ("WK LVDT's Limit Array"), binary string=w270, error in (no error)=w265) -> (value=w269:T22[])  [unwired: 2 in, 2 out]
        n124 = property on="LVDT's Limit Array" class="Arr (严格)"("Value"=w269) -> ()  [unwired: 2 in, 2 out]
      }
      frame "LVDT's Data Write to File" {
        n125 = Unbundle By Name(w278) -> ("paths.Base Path"=w277:path)
        n126 = property on="LVDT Part Type" class="Ring (严格)"() -> ("RingText.Text"=w279:string)  [unwired: 2 in, 2 out]
        n127 = call "get path to lvdt presets.vi"("product"=w279, "paths.Base Path"=w277) -> ("path"=w280:path)  [unwired: 9 in]
        n128 = property on="LVDT's Limit Array" class="Arr (严格)"() -> ("Value"=w288:T22[])  [unwired: 2 in, 2 out]
        n129 = Flatten To String(anything=w288) -> (data string=w282:string, error out=w281:errorcluster)  [unwired: 3 in, 1 out]
        n130 = call <vilib>:"Open Config Data.vi"("error in (no error)"=w281, "configuration file path"=w280) -> ("error out"=w283:errorcluster, "refnum"=w286:T56)  [unwired: 7 in, 1 out]
        n131 = call-poly <vilib>:"Write Key.vi"("section"="LVDT's Preset Data", "error in (no error)"=w283, "value"=w282, "key"=w279, "refnum"=w286) -> ("error out"=w284:errorcluster, "refnum out"=w285:T56)  [unwired: 4 in, 1 out]
        n132 = call <vilib>:"Close Config Data.vi"("error in (no error)"=w284, "refnum"=w285) -> ()  [unwired: 8 in, 2 out]
      }
      frame "LVDTs Read Data" {
        n133 = call <vilib>:"Set Busy.vi"() -> ("error out"=w292:errorcluster)  [unwired: 10 in, 1 out]
        n134 = Unbundle By Name(w302) -> ("rs232 port map.LVDT Unit"=w298:refnum<visa-resource-name>, "rs232 port map.LVDT Unit"=w291:refnum<visa-resource-name>)  [unwired: 1 out]
        n135 = Empty String/Path?(string/path=w298) -> (empty?=w293:bool)
        n136 = local read "LVDT's Limit Array"() -> (w301:T22[])
        n137 = call "Read LVDT's Data.vi"("Desired Decimal Points"="Desired Decimal Points", "truncate instead of round"="truncate instead of round", "error in"=w292, "rs232?"=w293, "LVDT's Com Port"=w291) -> ("error out"=w297:errorcluster, "Array"=w307:sgl[])  [unwired: 5 in]
        n138 = for {
          tunnel: w301 -> [w311] mode=indexing
          tunnel: w307 -> [w310] mode=indexing
          tunnel: [w309] -> w300 mode=indexing
          shift-right: [w308] -> w294
          shift-left: w297 -> [w308]
          n139 = Bundle By Name(cluster=w311, "Upper Limit"=w310) -> (w309:T22)
        }
        n140 = local write "LVDT's Limit Array"(w300) -> ()
        n141 = call <vilib>:"Clear Errors.vi"("error in (no error)"=w294) -> ("error out"=w299:errorcluster)  [unwired: 5 in, 1 out]
        n142 = call <vilib>:"Unset Busy.vi"("error in (no error)"=w299) -> ()  [unwired: 10 in, 1 out]
        n143 = call "Insert Multiple Events.vi"("Events to Insert"=string[] [] ("event queue out"), "Event queue in"=w306) -> ("Event queue out"=w305:string[])  [unwired: 5 in]
      }
      frame "LVDTs Write Data" {
        n144 = call <vilib>:"Set Busy.vi"() -> ("error out"=w314:errorcluster)  [unwired: 10 in, 1 out]
        n145 = local read "LVDT's Limit Array"() -> (w320:T22[])
        n146 = Unbundle By Name(w321) -> ("rs232 port map.LVDT Unit"=w323:refnum<visa-resource-name>)
        n147 = for {
          tunnel: w320 -> [w332] mode=indexing
          shift-right: [w328] -> w316
          shift-left: dbl[] [] -> [w327]
          shift-right: [w326] -> w317
          shift-left: i32[] [] -> [w325]
          i -> [w329]
          n148 = Unbundle By Name(w332) -> ("Check"=w331:bool, "Lower Limit"=w330:dbl)
          n149 = case shown="真" w331 {
            tunnel: w330 -> [_ w340]
            tunnel: w329 -> [_ w337]
            tunnel: [w334 w339] -> w328
            tunnel: w327 -> [w334 w338]
            tunnel: [w333 w336] -> w326
            tunnel: w325 -> [w333 w335]
            frame False {
            }
            frame True {
              n150 = Build Array (concatenate)(w335, w337) -> (w336:i32[])
              n151 = Build Array (concatenate)(w338, w340) -> (w339:dbl[])
            }
          }
        }
        n152 = call-poly "VISA Configure Serial Port"("VISA resource name"=w323, "error in (no error)"=w314) -> ("VISA resource name out"=w315:refnum<visa-resource-name>)  [unwired: 12 in, 1 out]
        n153 = call "Manual Set LVDT's.vi"("LVDT Numbers"=w317, "Data"=w316, "LVDT's 1"=w315) -> ("Error"=w313:errorcluster)  [unwired: 7 in, 1 out]
        n154 = call <vilib>:"Clear Errors.vi"("error in (no error)"=w313) -> ("error out"=w312:errorcluster)  [unwired: 5 in, 1 out]
        n155 = call <vilib>:"Unset Busy.vi"("error in (no error)"=w312) -> ()  [unwired: 10 in, 1 out]
      }
      frame "Print Audit St Barcode" {
        n156 = Unbundle By Name(w342) -> ("paths.Base Path"=w341:path)
        n157 = call "Log In 2.0.vi"("Program Root Path"=w341) -> ("Cancelled"=w343:bool, "passed"=w345:bool)  [unwired: 6 in, 3 out]
        n158 = Compound Arithmetic op=AND(w345, invert w343) -> (w344:bool)
        n159 = case shown="假" w344 {
          tunnel: w341 -> [_ w348]
          frame False {
          }
          frame True {
            n160 = property on="Barcode Print Part Type" class="Ring (严格)"() -> ("Strings []"=w357:string[], "Value"=w358:u16)  [unwired: 2 in, 2 out]
            n161 = Index Array(array=w357, index=w358) -> (element=w349:string)
            n162 = call "get path to audit barcode formats.vi"("product"=w349, "paths.Base Path"=w348) -> ("path"=w363:path)  [unwired: 9 in]
            n163 = call <vilib>:"Check if File or Folder Exists.vi"("path"=w363) -> ("error out"=w362:errorcluster, "file or folder exists?"=w360:bool, "dup path"=w361:path)  [unwired: 8 in]
            n164 = case shown="真" w360 {
              tunnel: w361 -> [_ w370]
              tunnel: w362 -> [w366 w369]
              tunnel: [w366 w368] -> w359
              tunnel: [w365 w367] -> w364
              frame False {
                w365 = T45[] []  # Frame Barcode Formats
              }
              frame True {
                n165 = call "read barcode formats.vi"("error in"=w369, "configuration file path"=w370) -> ("error out"=w368:errorcluster, "Frame Barcode Formats"=w367:T45[])  [unwired: 8 in]
              }
            }
            n166 = call "Barcode Print.vi"("part type"=w349, "Manual?"=TRUE, "error in"=w359, "Part History Number"="PHN:", "Plant Number"="Line Number", "Customer Number"="Customer Number:", "Color"="Sunshade Color", "Serial Number"="Serial Number:", "Inalfa Part Number"="IRS Number:", "Frame Barcode Formats"=w364) -> ()  [unwired: 1 in, 1 out]
          }
        }
      }
      frame "Print St 60 Barcode" {
        n167 = Unbundle By Name(w381) -> ("paths.Base Path"=w379:path)
        n168 = call "Log In 2.0.vi"("Program Root Path"=w379) -> ("User Name Out"=w376:string, "Cancelled"=w383:bool, "passed"=w375:bool)  [unwired: 6 in, 2 out]
        n169 = Compound Arithmetic op=AND(w375, invert w383) -> (w382:bool)
        n170 = case shown="真" w382 {
          tunnel: w379 -> [_ w387]
          tunnel: [_ "Module Serial Number"] -> w372
          frame False {
          }
          frame True {
            n171 = property on="Barcode Print Part Type" class="Ring (严格)"() -> ("Strings []"=w402:string[], "Value"=w401:u16)  [unwired: 2 in, 2 out]
            n172 = Index Array(array=w402, index=w401) -> (element=w390:string)
            n173 = call "get path to barcode formats.vi"("product"=w390, "paths.Base Path"=w387) -> ("path"=w397:path)  [unwired: 9 in]
            n174 = call <vilib>:"Check if File or Folder Exists.vi"("path"=w397) -> ("error out"=w400:errorcluster, "file or folder exists?"=w398:bool, "dup path"=w399:path)  [unwired: 8 in]
            n175 = case shown="假" w398 {
              tunnel: w399 -> [_ w408]
              tunnel: w400 -> [w404 w407]
              tunnel: [w404 w406] -> w389
              tunnel: [T45[] [] ("Frame Barcode Formats") w405] -> w393
              frame False {
              }
              frame True {
                n176 = call "read barcode formats.vi"("error in"=w407, "configuration file path"=w408) -> ("error out"=w406:errorcluster, "Frame Barcode Formats"=w405:T45[])  [unwired: 8 in]
              }
            }
            n177 = local read "Line Number"() -> (w388:u8)
            n178 = call "Barcode Print.vi"("part type"=w390, "Manual?"=TRUE, "error in"=w389, "Part History Number"="TLL/PHN", "Plant Number"=w388, "Customer Number"="Customer Number", "Color"="Color Name", "Serial Number"="Module Serial Number", "Inalfa Part Number"="Inalfa Part Number", "Frame Barcode Formats"=w393) -> ()  [unwired: 1 in, 1 out]
          }
        }
        n179 = Boolean To (0,1)(Boolean=w375) -> (0, 1=w373:i16)
        n180 = Number To Decimal String(number=w373) -> (decimal integer string=w374:string)  [unwired: 1 in]
        n181 = Build Path(base path=w379, name or relative path="System\\manual bc print log.txt") -> (appended path=w378:path)
        n182 = Build Array(w376, w374, w372) -> (w371:string[])
        n183 = call-poly <vilib>:"Write To Spreadsheet File.vi"("append to file? (new file:F)"=TRUE, "1D data"=w371, "file path (dialog if empty)"=w378) -> ()  [unwired: 5 in, 1 out]
      }
      frame "Re-Initialize PS Port" {
        n184 = Unbundle By Name(w410) -> ("rs232 port map.PS Port"=w413:refnum<visa-resource-name>, "misc station config.power supply type"=w409:T20)
        n185 = case shown="\"Manual\"" w409 {
          tunnel: w413 -> [_ w419]
          tunnel: [_ w418] -> w411
          tunnel: w409 -> [_ w417]
          frame "Manual" {
            n186 = One Button Dialog(message="The  power supply doesn't support Re-Initialize PS Port online in manual mode") -> ()  [unwired: 1 in, 1 out]
          }
          frame Default {
            n187 = call "EOL Initialize Power Supplies.vi"("power supply model"=w417, "VISA resource name"=w419) -> ("error out"=w418:errorcluster)  [unwired: 9 in]
          }
        }
        n188 = Bundle By Name(cluster=w415, "error out"=w411) -> (w412:T41)
      }
      frame "Send Inalfa SCU Message" {
        n189 = Unbundle By Name(w431) -> ("LIN INFO.Toolkit Type"=w432:enum16{"Inalfa LIN", "ADCS LIN", "TS LIN"}, "LIN INFO.NAD"=w433:u8, "LIN INFO.Inalfa LIN"=w449:T32)
        n190 = Unbundle By Name(w431) -> ("LIN INFO.TS LIN"=w422:T57, "LIN INFO.ADCS LIN"=w430:T33)
        n191 = local read "Choose Sequence"() -> (w450:T38)
        n192 = property on="Part Type" class="Ring (严格)"() -> ("RingText.Text"=w428:string)  [unwired: 2 in, 2 out]
        n193 = property on="Multicolumn Listbox" class="MCListbox (严格)"() -> ("ItemNames"=w421:string[][])  [unwired: 2 in, 2 out]
        n194 = Unbundle By Name(w425) -> ("Sequence State in"=w426:T40)
        n195 = case shown="\"ADCS LIN\"" w432 {
          tunnel: w450 -> [w470 w497 w534]
          tunnel: w449 -> [w469 _ _]
          tunnel: "Position" -> [w468 w494 w531]
          tunnel: "Vent Cycles" -> [w467 w493 w530]
          tunnel: "Slide Cycles" -> [w466 w492 w529]
          tunnel: "Tx2" -> [w465 w491 w528]
          tunnel: [w464 w484 w521] -> w444
          tunnel: [w463 w483 w520] -> w443
          tunnel: [w462 w482 w519] -> w442
          tunnel: [w461 w478 w515] -> _
          tunnel: [w460 w498 w535] -> w441
          tunnel: [w459 w479 w516] -> w439
          tunnel: [w458 w480 w517] -> w438
          tunnel: [w457 w481 w518] -> w437
          tunnel: "Rx2" -> [w456 w490 w527]
          tunnel: "Tx3" -> [w455 w489 w526]
          tunnel: "BYD Teach" -> [w454 w495 w532]
          tunnel: w433 -> [w453 _ _]
          tunnel: w428 -> [_ w500 w536]
          tunnel: w430 -> [_ w499 _]
          tunnel: T47 {"Slide Cycles"=0, "Vent Cycles"=0, "String"="", "Tx Bytes"=[], "Rx Bytes"=[], "Only Tx1 Bytes"=[], "Go to Position"=0, "Check Glass Position"=0, "Checkgalss"=TRUE, "Check Sunshade Position"=0, "Checksunshade"=TRUE} ("LIN show messages") -> [_ w496 w533]
          tunnel: [_ w486 w523] -> w427
          tunnel: w426 -> [w452 w476 w513]
          tunnel: [w452 w475 w512] -> w423
          tunnel: w422 -> [_ _ w511]
          tunnel: w421 -> [_ w472 w508]
          tunnel: [w451 w471 w501] -> w420
          frame "Inalfa LIN", Default {
            n196 = call "Inalfa SCU_Manual_LIN Message.vi"("Choose Sequence"=w470, "LIN Device"=w469, "Position"=w468, "Vent Cycles"=w467, "Slide Cycles"=w466, "Tx"=w465, "Only Tx"=w455, "Rx"=w456, "String"=w454, "NAD"=w453) -> ("glass position"=w457:u16, "TxRx Data"=w451:string[][], "sunshade position"=w458:u16, "Response Good?"=w460:bool, "Software Level"=w464:string, "Hardware Level"=w463:string, "Calfile Level"=w462:string, "Glass Slide Cycle"=w459:u16, "Rx2"=w461:u8[])  [unwired: 1 in]
          }
          frame "ADCS LIN" {
            n197 = Bundle By Name(cluster=w496, "String"=w495, "Only Tx1 Bytes"=w489, "Go to Position"=w494, "Vent Cycles"=w493, "Slide Cycles"=w492, "Tx Bytes"=w491, "Rx Bytes"=w490) -> (w488:T47)
            n198 = Flatten To String(anything=w488) -> (data string=w487:string)  [unwired: 3 in, 2 out]
            n199 = call <vilib>:"Inalfa ADCS LIN.vi"("seq in"=w497, "Sequence State.Step Data String"=w487, "manual control?"=TRUE, "ADCS_LIN info"=w499, "Mode type"=w500, "Sequence State in"=w476) -> ("Sequence State out"=w475:T40, "Manual Data"=w485:T58, "error description"=w486:string, "pass?"=w498:bool, "LIN.LINRecData"=w478:u8[], "LIN.LINbyteLog"=w474:string)  [unwired: 3 in, 5 out]
            n200 = Spreadsheet String To Array(format string="" ("分隔符(Tab)"), spreadsheet string=w474, array type (2D Dbl)=w472) -> (array=w471:string[][])  [unwired: 1 in]
            n201 = Unbundle By Name(w485) -> ("SW"=w484:string, "HW"=w483:string, "Cal"=w482:string, "Cycle.Slide"=w479:u16, "Hall.Rollo"=w480:i16, "Hall.Glass"=w481:i16)
          }
          frame "TS LIN" {
            n202 = Bundle By Name(cluster=w533, "String"=w532, "Only Tx1 Bytes"=w526, "Go to Position"=w531, "Vent Cycles"=w530, "Slide Cycles"=w529, "Tx Bytes"=w528, "Rx Bytes"=w527) -> (w525:T47)
            n203 = Flatten To String(anything=w525) -> (data string=w524:string)  [unwired: 3 in, 2 out]
            n204 = call <vilib>:"Inalfa TS LIN.vi"("seq in"=w534, "Sequence State.Step Data String"=w524, "manual control?"=TRUE, "Ts_LIN info"=w511, "Mode type"=w536, "Sequence State in"=w513) -> ("Sequence State out"=w512:T40, "Manual Data"=w522:T58, "Error Description"=w523:string, "pass?"=w535:bool, "LINRecData"=w515:u8[], "LIN.LINbyteLog"=w509:string)  [unwired: 3 in, 5 out]
            n205 = Spreadsheet String To Array(format string="" ("分隔符(Tab)"), spreadsheet string=w509, array type (2D Dbl)=w508) -> (array=w507:string[][])  [unwired: 1 in]
            n206 = Unbundle By Name(w522) -> ("SW"=w521:string, "HW"=w520:string, "Cal"=w519:string, "Cycle.Slide"=w516:u16, "Hall.Rollo"=w517:i16, "Hall.Glass"=w518:i16)
            n207 = Delete From Array(array=w507, length=2 ("长度"), index (col)=1 ("禁用的索引 (列)")) -> (array with subset deleted=w504:string[][])  [unwired: 1 in, 1 out]
            n208 = Delete From Array(array=w504, length=1 ("长度"), index (col)=2 ("禁用的索引 (列)")) -> (array with subset deleted=w501:string[][])  [unwired: 1 in, 1 out]
          }
        }
        "Software Level" <- w444
        "Hardware Level" <- w443
        "Calfile Level" <- w442
        "sunshade position" <- w438
        "glass position" <- w437
        "slide cycle" <- w439
        n209 = Bundle By Name(cluster=w425, "Sequence State in"=w423) -> (w424:T41)
        n210 = property on="Multicolumn Listbox" class="MCListbox (严格)"("ItemNames"=w420) -> ()  [unwired: 2 in, 2 out]
        n211 = property on="String" class="Str"("Value"=w427) -> ()  [unwired: 2 in, 2 out]
        n212 = local write "Recive？"(w441) -> ()
      }
      frame "Hold EOL Session" {
        n213 = Unbundle By Name(w553) -> ("LIN INFO.Toolkit Type"=w550:enum16{"Inalfa LIN", "ADCS LIN", "TS LIN"}, "LIN INFO.NAD"=w549:u8, "LIN INFO.Inalfa LIN"=w548:T32, "LIN INFO.ADCS LIN"=w552:T33, "LIN INFO.TS LIN"=w537:T57)
        n214 = Unbundle By Name(w542) -> ("Sequence State in"=w541:T40)
        n215 = Bundle By Name(cluster=w541, "Hold?"=TRUE) -> (w543:T40)
        n216 = property on="Part Type" class="Ring (严格)"() -> ("RingText.Text"=w540:string)  [unwired: 2 in, 2 out]
        n217 = case shown="\"ADCS LIN\"" w550 {
          tunnel: w552 -> [_ w565 _]
          tunnel: "Hold EOL session" -> [w555 w564 w573]
          tunnel: w549 -> [w556 _ _]
          tunnel: w548 -> [w557 _ _]
          tunnel: w543 -> [w554 w563 w572]
          tunnel: w540 -> [_ w562 w571]
          tunnel: [_ w560 w566] -> w539
          tunnel: [w554 w558 w569] -> w538
          tunnel: w537 -> [_ _ w568]
          frame "Inalfa LIN", Default {
            n218 = call "Inalfa SCU_Manual_LIN Message.vi"("Choose Sequence"=w555, "LIN Device"=w557, "NAD"=w556) -> ()  [unwired: 8 in, 9 out]
          }
          frame "ADCS LIN" {
            n219 = call <vilib>:"Inalfa ADCS LIN.vi"("seq in"=w564, "manual control?"=TRUE, "ADCS_LIN info"=w565, "Mode type"=w562, "Sequence State in"=w563) -> ("Sequence State out"=w558:T40, "Manual Data"=w561:T58)  [unwired: 4 in, 9 out]
            n220 = Unbundle By Name(w561) -> ("Hold？"=w560:bool)
          }
          frame "TS LIN" {
            n221 = call <vilib>:"Inalfa TS LIN.vi"("seq in"=w573, "manual control?"=TRUE, "Ts_LIN info"=w568, "Mode type"=w571, "Sequence State in"=w572) -> ("Sequence State out"=w569:T40, "Manual Data"=w567:T58)  [unwired: 4 in, 9 out]
            n222 = Unbundle By Name(w567) -> ("Hold？"=w566:bool)
          }
        }
        "Hold？" <- w539
        n223 = Tick Count (ms)() -> (millisecond timer value=w545:u32)
        n224 = Bundle By Name(cluster=w542, "millisecond timer value"=w545, "Sequence State in"=w538) -> (w546:T41)
      }
      frame "Send List Msg" {
        n225 = Unbundle By Name(w593) -> ("LIN INFO.Toolkit Type"=w591:enum16{"Inalfa LIN", "ADCS LIN", "TS LIN"}, "LIN INFO.NAD"=w590:u8, "LIN INFO.Inalfa LIN"=w589:T32, "LIN INFO.ADCS LIN"=w592:T33, "LIN INFO.TS LIN"=w576:T57)
        n226 = Unbundle By Name(w579) -> ("Sequence State in"=w580:T40)
        n227 = property on="Message List" class="MCListbox (严格)"() -> ("ItemNames"=w585:string[][])  [unwired: 2 in, 2 out]
        n228 = Index Array(array=w585, index (row)="Message List", index (col)=0 ("disabled index (col)")) -> (element=w583:string)
        n229 = property on="Part Type" class="Ring (严格)"() -> ("RingText.Text"=w582:string)  [unwired: 2 in, 2 out]
        n230 = property on="Multicolumn Listbox" class="MCListbox (严格)"() -> ("ItemNames"=w575:string[][])  [unwired: 2 in, 2 out]
        n231 = case shown="\"Inalfa LIN\", 默认" w591 {
          tunnel: w592 -> [_ w611 _]
          tunnel: w583 -> [w597 w610 w629]
          tunnel: w590 -> [w598 _ _]
          tunnel: w589 -> [w599 _ _]
          tunnel: [_ w609 w628] -> _
          tunnel: [w596 w608 w627] -> w587
          tunnel: w582 -> [_ w607 w626]
          tunnel: w580 -> [w595 w605 w624]
          tunnel: [w595 w604 w623] -> w577
          tunnel: w576 -> [_ _ w622]
          tunnel: w575 -> [_ w601 w621]
          tunnel: [w594 w600 w612] -> w574
          frame "Inalfa LIN", Default {
            n232 = call "Inalfa SCU_Manual_LIN Message.vi"("Choose Sequence"=w597, "LIN Device"=w599, "NAD"=w598) -> ("TxRx Data"=w594:string[][], "Response Good?"=w596:bool)  [unwired: 8 in, 7 out]
          }
          frame "ADCS LIN" {
            n233 = call <vilib>:"Inalfa ADCS LIN.vi"("seq in"=w610, "manual control?"=TRUE, "ADCS_LIN info"=w611, "Mode type"=w607, "Sequence State in"=w605) -> ("Sequence State out"=w604:T40, "error description"=w609:string, "pass?"=w608:bool, "LIN.LINbyteLog"=w602:string)  [unwired: 4 in, 7 out]
            n234 = Spreadsheet String To Array(format string="" ("分隔符(Tab)"), spreadsheet string=w602, array type (2D Dbl)=w601) -> (array=w600:string[][])  [unwired: 1 in]
          }
          frame "TS LIN" {
            n235 = call <vilib>:"Inalfa TS LIN.vi"("seq in"=w629, "manual control?"=TRUE, "Ts_LIN info"=w622, "Mode type"=w626, "Sequence State in"=w624) -> ("Sequence State out"=w623:T40, "Error Description"=w628:string, "pass?"=w627:bool, "LIN.LINbyteLog"=w620:string)  [unwired: 4 in, 7 out]
            n236 = Spreadsheet String To Array(format string="" ("分隔符(Tab)"), spreadsheet string=w620, array type (2D Dbl)=w621) -> (array=w613:string[][])  [unwired: 1 in]
            n237 = Delete From Array(array=w613, length=2 ("长度"), index (col)=1 ("禁用的索引 (列)")) -> (array with subset deleted=w616:string[][])  [unwired: 1 in, 1 out]
            n238 = Delete From Array(array=w616, length=1 ("长度"), index (col)=2 ("禁用的索引 (列)")) -> (array with subset deleted=w612:string[][])  [unwired: 1 in, 1 out]
          }
        }
        n239 = Bundle By Name(cluster=w579, "Sequence State in"=w577) -> (w578:T41)
        n240 = local write "Recive？"(w587) -> ()
        n241 = property on="String" class="Str"("Value"="" ("String")) -> ()  [unwired: 2 in, 2 out]
        n242 = property on="Multicolumn Listbox" class="MCListbox (严格)"("ItemNames"=w574) -> ()  [unwired: 2 in, 2 out]
      }
      frame "Set Voltage" {
        n243 = Unbundle By Name(w633) -> ("rs232 port map.PS Port"=w632:refnum<visa-resource-name>, "misc station config.power supply type"=w630:T20)
        n244 = case shown="\"Manual\"" w630 {
          tunnel: w632 -> [_ w640]
          tunnel: w630 -> [_ w638]
          tunnel: "Output Voltage" -> [_ w637]
          frame "Manual" {
            n245 = One Button Dialog(message="The  power supply doesn't support setting voltage online in manual mode") -> ()  [unwired: 1 in, 1 out]
          }
          frame Default {
            n246 = call "EOL Initialize Power Supplies.vi"("Volt Limit"=w637, "power supply model"=w638, "No. of Power Supplies"=1 ("Number of Power Supplies"), "VISA resource name"=w640) -> ()  [unwired: 7 in, 1 out]
          }
        }
      }
      frame "Upload Message List" {
        n247 = Unbundle By Name(w641) -> ("paths.Base Path"=w643:path, "misc status.Part Setup.Communication Type"=w642:T27)
        n248 = case shown="默认" w642 {
          selector: w642 -> [_ w646]
          tunnel: w643 -> [_ w651]
          frame "P42M-Continental" {
          }
          frame Default {
            n249 = case shown="\"SnT LIN\"" w646 {
              tunnel: ["System\\Communication Message List\\CAN Messages INI File.txt" "System\\Communication Message List\\RS232 Messages INI File.txt" "System\\Communication Message List\\RS232 Messages INI File.txt" "System\\Communication Message List\\RS232 Messages INI File.txt" "System\\Communication Message List\\RS232 Messages INI File.txt" "System\\Communication Message List\\SnT Messages INI File.txt" "System\\Communication Message List\\K Line Messages INI File.txt" "System\\Communication Message List\\Robel CAN Messages INI File.txt" "System\\Communication Message List\\Spare 1 Messages INI File.txt" "System\\Communication Message List\\Spare 2 Messages INI File.txt" "System\\Communication Message List\\Spare 3 Messages INI File.txt"] -> w650
              frame "CAN" {
              }
              frame "RS 232" {
              }
              frame "RS 232 LIN" {
              }
              frame "GM LIN" {
              }
              frame "None" {
              }
              frame "SnT LIN" {
              }
              frame "K Line" {
              }
              frame "Robel CAN" {
              }
              frame "P42M-Continental" {
              }
              frame "Inalfa SCU LIN" {
              }
              frame "Spare 3" {
              }
            }
            n250 = Build Path(base path=w651, name or relative path=w650) -> (appended path=w648:path)
            n251 = call <vilib>:"Check if File or Folder Exists.vi"("path"=w648) -> ("file or folder exists?"=w649:bool, "dup path"=w647:path)  [unwired: 8 in, 1 out]
            n252 = case shown="假" w649 {
              tunnel: w647 -> [_ w653]
              frame False {
                n253 = property on="String" class="Str"("Value"="No Message List Exists for this Communication Type" ("String")) -> ()  [unwired: 2 in, 2 out]
              }
              frame True {
                n254 = call-poly <vilib>:"Read From Spreadsheet File.vi"("file path (dialog if empty)"=w653) -> ("all rows"=w657:string[][])  [unwired: 6 in, 4 out]
                n255 = Delete From Array(array=w657, length=1, index (row)=0) -> (array with subset deleted=w654:string[][])  [unwired: 1 in, 1 out]
                n256 = property on="Message List" class="MCListbox (严格)"("ItemNames"=w654) -> ()  [unwired: 2 in, 2 out]
              }
            }
          }
        }
      }
      frame "Write RSLinx Write Data" {
        n257 = Unbundle By Name(w670) -> ("Config Info"=w671:T34)
        n258 = call "Config Info Get.vi"("Config Info"=w671) -> ("PLC Comms"=w669:T49)  [unwired: 7 in, 3 out]
        n259 = case shown="\"RSLinx Tags Write\"" w672 {
          tunnel: w669 -> [_ w682]
          frame "Analog and Digital IO", Default {
          }
          frame "RSLinx Tags Write" {
            w675 = errorcluster {"status"=FALSE, "code"=0, "source"=""} ("error out")
            n260 = Unbundle By Name(w682) -> ("PLC bool write Tags"=w681:T53, "PLC string write Tags"=w680:T55)
            n261 = Cluster To Array(cluster=w681) -> (array=w679:T51[])
            n262 = Cluster To Array(cluster=w680) -> (array=w678:T51[])
            n263 = property on="RSLinx Write Tag Boolean Array Data" class="Arr (严格)"() -> ("Index Values"=w684:u32[])  [unwired: 2 in, 2 out]
            n264 = property on="RSLinx Write Tag String Array Data" class="Arr (严格)"() -> ("Index Values"=w683:u32[])  [unwired: 2 in, 2 out]
            n265 = for {
              tunnel: w679 -> [w700] mode=indexing
              tunnel: "RSLinx Write Tag Boolean Array Data" -> [w697] mode=indexing
              shift-right: [w698] -> _
              shift-left: w675 -> [w699]
              n266 = Unbundle By Name(w700) -> ("Tag Name"=w701:string)
              n267 = Empty String/Path?(string/path=w701) -> (empty?=w702:bool)
              n268 = case shown="假" w702 {
                tunnel: w697 -> [w704 _]
                tunnel: w700 -> [w707 _]
                tunnel: w699 -> [w706 w708]
                tunnel: [w705 w708] -> w698
                frame False {
                  n269 = call "plc write bool.vi"("error in"=w706, "value"=w704, "addr,tag"=w707) -> ("error out"=w705:errorcluster)  [unwired: 8 in]
                  n270 = Wait Until Next ms Multiple(millisecond multiple=u32 1) -> ()  [unwired: 1 out]
                }
                frame True {
                }
              }
            }
            n271 = for {
              tunnel: w678 -> [w685] mode=indexing
              tunnel: "RSLinx Write Tag String Array Data" -> [w690] mode=indexing
              shift-right: [w687] -> _
              shift-left: w675 -> [w686]
              n272 = Unbundle By Name(w685) -> ("Tag Name"=w689:string)
              n273 = Empty String/Path?(string/path=w689) -> (empty?=w688:bool)
              n274 = case shown="假" w688 {
                tunnel: w690 -> [w692 _]
                tunnel: [w695 w696] -> w687
                tunnel: w686 -> [w694 w696]
                tunnel: w685 -> [w693 _]
                frame False {
                  n275 = call "plc write string.vi"("error in"=w694, "value"=w692, "addr,tag"=w693) -> ("error out"=w695:errorcluster)  [unwired: 8 in]
                  n276 = Wait Until Next ms Multiple(millisecond multiple=u32 1) -> ()  [unwired: 1 out]
                }
                frame True {
                }
              }
            }
            n277 = property on="RSLinx Write Tag Boolean Array Names" class="Arr (严格)"("Index Values"=w684) -> ()  [unwired: 2 in, 2 out]
            n278 = property on="RSLinx Write Tag String Array Names" class="Arr (严格)"("Index Values"=w683) -> ()  [unwired: 2 in, 2 out]
          }
        }
      }
      frame "ECU Bootup Delay" {
        n279 = Wait (ms)(milliseconds to wait=u32 500) -> ()  [unwired: 1 out]
      }
      frame "Turn Power On" {
        # "***done manually"
      }
      frame "Check Sequence" {
      }
      frame "Turn RAP Off" {
        n280 = Unbundle By Name(w720) -> ("DO Task"=w719:refnum<k21>)
        n281 = case shown="假" w721 {
          tunnel: w719 -> [w724 _]
          frame False {
            n282 = Bundle By Name(cluster=T42 {"Status"=FALSE, "Global DO Ch"=enum."Battery"} ("Cluster"), "Status"=FALSE, "Global DO Ch"=EOL_Global_Digital_Output_Control."IGN High") -> (w728:T42)
            n283 = Build Array(w728) -> (w726:T42[])
            n284 = call "EOL Digital Outputs v3.vi"("task/channels in"=w724, "DO Status"=w726, "Mode"=T44."Write") -> ()  [unwired: 7 in, 2 out]
          }
          frame True {
          }
        }
      }
      frame "Turn RAP On" {
        n285 = Unbundle By Name(w732) -> ("DO Task"=w731:refnum<k21>)
        n286 = case shown="假" w733 {
          tunnel: w731 -> [w736 _]
          frame False {
            n287 = Bundle By Name(cluster=T42 {"Status"=FALSE, "Global DO Ch"=enum."Battery"} ("Cluster"), "Status"=TRUE, "Global DO Ch"=EOL_Global_Digital_Output_Control."IGN High") -> (w740:T42)
            n288 = Build Array(w740) -> (w738:T42[])
            n289 = call "EOL Digital Outputs v3.vi"("task/channels in"=w736, "DO Status"=w738, "Mode"=T44."Write") -> ()  [unwired: 7 in, 2 out]
          }
          frame True {
          }
        }
      }
      frame "Read PMAC" {
        n290 = Unbundle By Name(w746) -> ("rs232 port map.PMAC"=w744:refnum<visa-resource-name>)
        n291 = flat-sequence {
          tunnel: [w752] -> w743
          tunnel: w744 -> [w752]
          frame #0 {
            n292 = Wait (ms)(milliseconds to wait=u32 500) -> ()  [unwired: 1 out]
          }
        }
        n293 = property class="Instr"(reference=w743) -> (reference out=w749:refnum<visa-resource-name>, "Serial Settings:Number of Bytes at Serial Port"=w750:u32)  [unwired: 1 in, 1 out]
        n294 = VISA Read(VISA resource name=w749, byte count=w750) -> (read buffer=w747:string)  [unwired: 1 in, 3 out]
        "PMAC Reading 2" <- w747
        n295 = Empty String/Path?(string/path=w747) -> (empty?=w748:bool)
        n296 = case shown="假" w748 {
          tunnel: w747 -> [w756 _]
          frame False {
            n297 = String Subset(string=w756, offset (0)=8) -> (substring=w760:string)  [unwired: 1 in]
            n298 = String Subset(string=w756, offset (0)=2, length (rest)=4 ("length (rest)")) -> (substring=w757:string)
            n299 = Match Pattern(string=w760, regular expression=" ") -> (before substring=→"PMAC Reading":string)  [unwired: 1 in, 3 out]
            n300 = Scan From String(input string=w757) -> (output 1=→"Reading Count":dbl)  [unwired: 4 in, 3 out]
          }
          frame True {
          }
        }
      }
      frame "Clear PMAC Buffer" {
        n301 = Unbundle By Name(w764) -> ("rs232 port map.PMAC"=w766:refnum<visa-resource-name>)
        n302 = VISA Write(VISA resource name=w766, write buffer="C\rNNN\rN\r\u001b\u001b" ("spreadsheet string")) -> ()  [unwired: 1 in, 3 out]
      }
    }
  }
  "main thread cluster out" <- w7
